vi "气密封测试.vi"() -> ()   [LabVIEW 2014]
uses:
  <vilib>/Instr/_visa.llb/VISA Flush IO Buffer Mask.ctl
  <vilib>/Utility/config.llb/NI_LVConfig.lvlib
  <vilib>/Utility/config.llb/Write Key (String).vi
  <vilib>/Utility/miscctls.llb/LVRowAndColumnTypeDef.ctl
  <vilib>/Utility/config.llb/Read Key (String).vi
  <vilib>/Instr/_visa.llb/VISA Configure Serial Port (Instr).vi
panel:
  in  "右扫码启动":bool
  in  "左扫码启动":bool
  in  "错误输入（无错误） 2":errorcluster caption="错误输入（无错误）"
  out "错误输出 4":errorcluster caption="错误输出"
  out "错误输出 3":errorcluster caption="错误输出"
  in  "错误输入（无错误）":errorcluster
  out "合格 2":bool
  out "StepCode 2":u16
  out "Ready 2":bool
  out "右合格":bool
  out "替换数量 2":i32
  out "结果 2":string
  in  "合格次数 2":u16
  out "泄漏单位 2":string
  out "压力单位 2":string
  in  "检测次数 2":u16
  in  "合格状态右":dbl=2.0
  out "StatusResults 2":u16 format="%b"
  out "LeakUnit 2":u16(ring) items=["ml/min"=51000, "cm3/s"=0, "cm3/min"=1000, "cm3/h"=2000, "mm3/h"=3000, "CalibartedPascal"=4000, "Pa"=6000, "Bar"=11000, "Kpa"=12000, "PSI"=13000, "Mbar"=14000, "Mpa"=15000, "Inch3/s"=46000, "Inch3/min"=47000, "Inch3/hour"=48000]
  out "PressureUnit 2":u16(ring) items=["cm3/s"=0, "cm3/min"=1000, "cm3/h"=2000, "mm3/h"=3000, "CalibartedPascal"=4000, "Pa"=6000, "Bar"=11000, "Kpa"=12000, "PSI"=13000, "Mbar"=14000, "Mpa"=15000, "Inch3/s"=46000, "Inch3/min"=47000, "Inch3/hour"=48000]
  out "ProgramNumber 2":u16
  out "结果压力 2":dbl
  out "结果漏率 2":dbl
  out "扫码信息 B":string
  out "开始启动仪器 2":bool
  out "开始启动仪器":bool
  in  "扫码选程序":bool=TRUE
  out "错误输出":errorcluster
  out "写入的字节":i32
  out "数值 2":i32
  in  "扫码流程":dbl
  out "左合格":bool
  out "合格":bool
  in  "合格次数":u16
  in  "检测次数":u16
  out "扫码信息A":string
  out "结果漏率":dbl
  out "结果压力":dbl
  out "替换数量":i32
  out "ATEQ程序号-1":i32
  in  "扫码关键词":u16(ring)
  in  "启动仪器":dbl
  out "ProgramNumber":u16
  in  "选项卡控件":enum32{"主页面", "设置"}(tab)
  in  "扫码开/关B":bool
  in  "扫码开/关A":bool
  in  "选择检验员B":u16(ring) items=["李红", "", "", "", "", "", "", "", "", "", "", "", "", "", "", "", "", "", "", "", "", "", "", "", "", "", "", "", "", "", "", "", "", "", ""]
  in  "选择产品型号B":u16(ring) items=["EV80", "E109", "", "", "", "", "", "", "", "", "", "", "", "", "", "", "", "", "", "", "", "", "", "", "", "", "", "", "", "", "", "", "", "", ""]
  in  "单腔/双腔A":bool
  out "最终结果A":bool
  in  "选择检验员A":u16(ring) items=["李红", "", "", "", "", "", "", "", "", "", "", "", "", "", "", "", "", "", "", "", "", "", "", "", "", "", "", "", "", "", "", "", "", "", ""]
  out "实时压力A":dbl
  out "实时漏率A":dbl
  in  "确定修改A":bool
  out "当前序号A":string
  in  "序号清零A":bool
  in  "修改当前序号A":string
  out "显示表格":string[][](table)
  in  "选择产品型号A":u16(ring) items=["EV80", "E109", "", "", "", "", "", "", "", "", "", "", "", "", "", "", "", "", "", "", "", "", "", "", "", "", "", "", "", "", "", "", "", "", ""]
  out "程序号":i32
  out "二维码A":string
  out "二维码B":string
  out "实时压力B":dbl
  out "实时漏率B":dbl
  out "最终结果B":bool
  in  "单腔/双腔B":bool
  in  "修改当前序号B":string
  in  "确定修改B":bool
  in  "序号清零B":bool
  out "当前序号B":string
  in  "表格控件":string[][](table)
  in  "确定按钮":bool
  in  "活动单元格:活动单元格":T1
  out "泄漏单位":string
  out "压力单位":string
  out "PressureUnit":u16(ring) items=["cm3/s"=0, "cm3/min"=1000, "cm3/h"=2000, "mm3/h"=3000, "CalibartedPascal"=4000, "Pa"=6000, "Bar"=11000, "Kpa"=12000, "PSI"=13000, "Mbar"=14000, "Mpa"=15000, "Inch3/s"=46000, "Inch3/min"=47000, "Inch3/hour"=48000]
  out "StatusResults":u16 format="%b"
  out "LeakUnit":u16(ring) items=["ml/min"=51000, "cm3/s"=0, "cm3/min"=1000, "cm3/h"=2000, "mm3/h"=3000, "CalibartedPascal"=4000, "Pa"=6000, "Bar"=11000, "Kpa"=12000, "PSI"=13000, "Mbar"=14000, "Mpa"=15000, "Inch3/s"=46000, "Inch3/min"=47000, "Inch3/hour"=48000]
  in  "合格状态左":dbl
  out "Ready":bool
  out "StepCode":u16
  out "结果":string
  # "气密性检测设备"
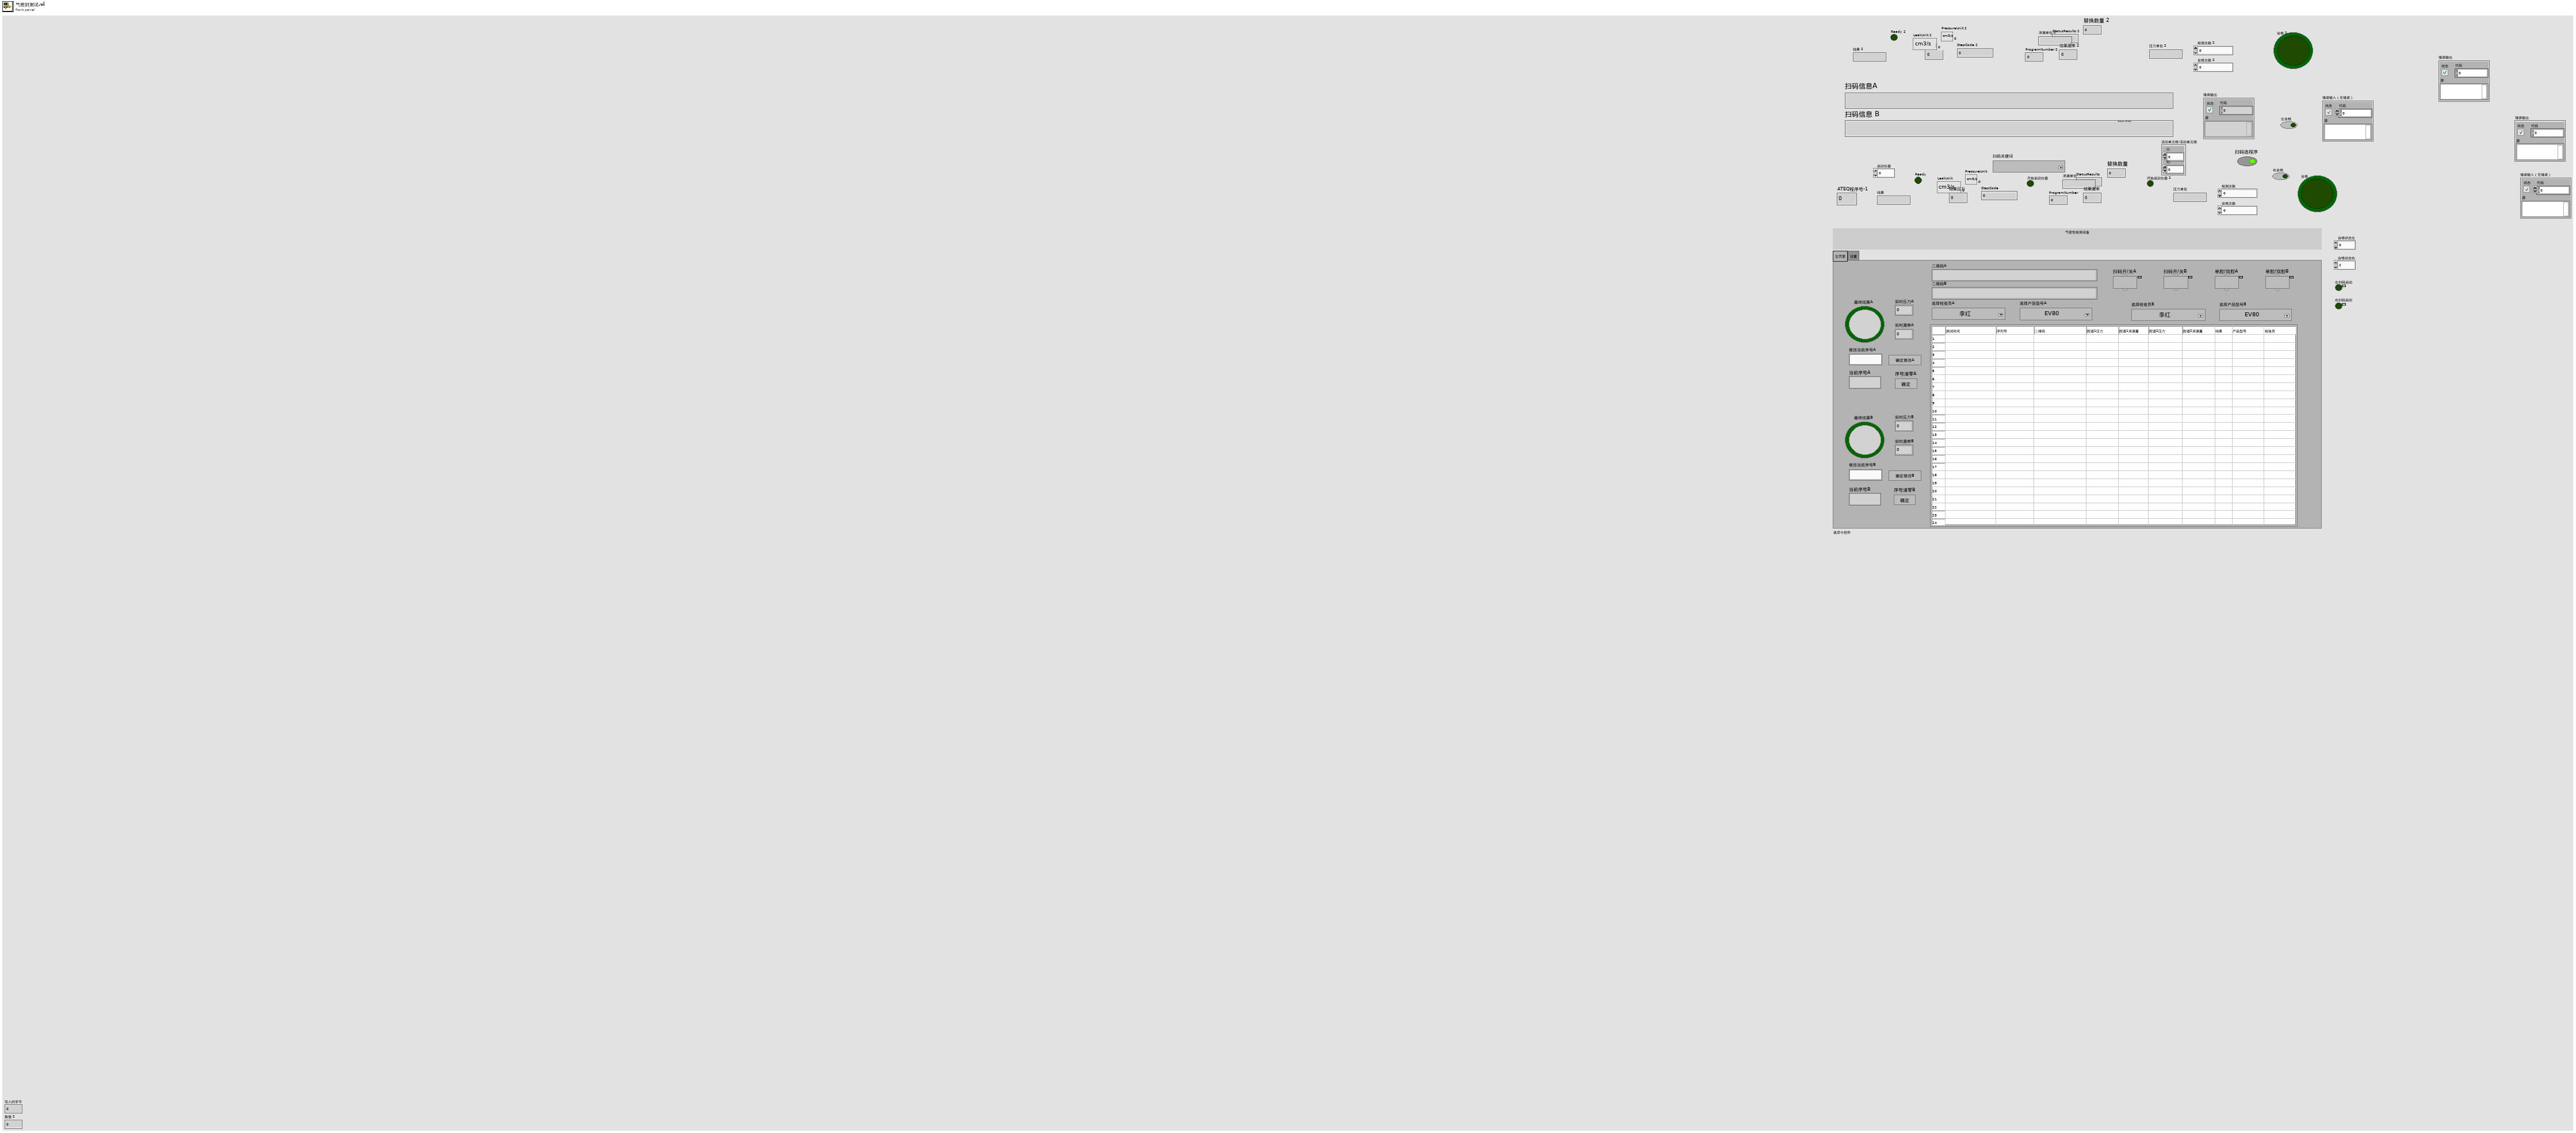
[diagram p1: front panel]
types:
  T1 = typedef "LVRowAndColumnTypeDef.ctl" = cluster{"Row":i32, "Column":i32}
  T2 = enum16{"Init", "Loop", "Write LOFF", "Write LON", "Read", "Exit", "Open", "Close"}
  T3 = typedef "NI_LVConfig.lvlib/Config Data RefNum.ctl" = refnum<k1>
  T4 = enum8{"Enabled", "Disabled", "Disabled and Grayed Out"}
  T5 = typedef "VISA Flush IO Buffer Mask.ctl" = u16
  T6 = enum16{"Standard", "Buffered", "CRLF", "Immediate"}
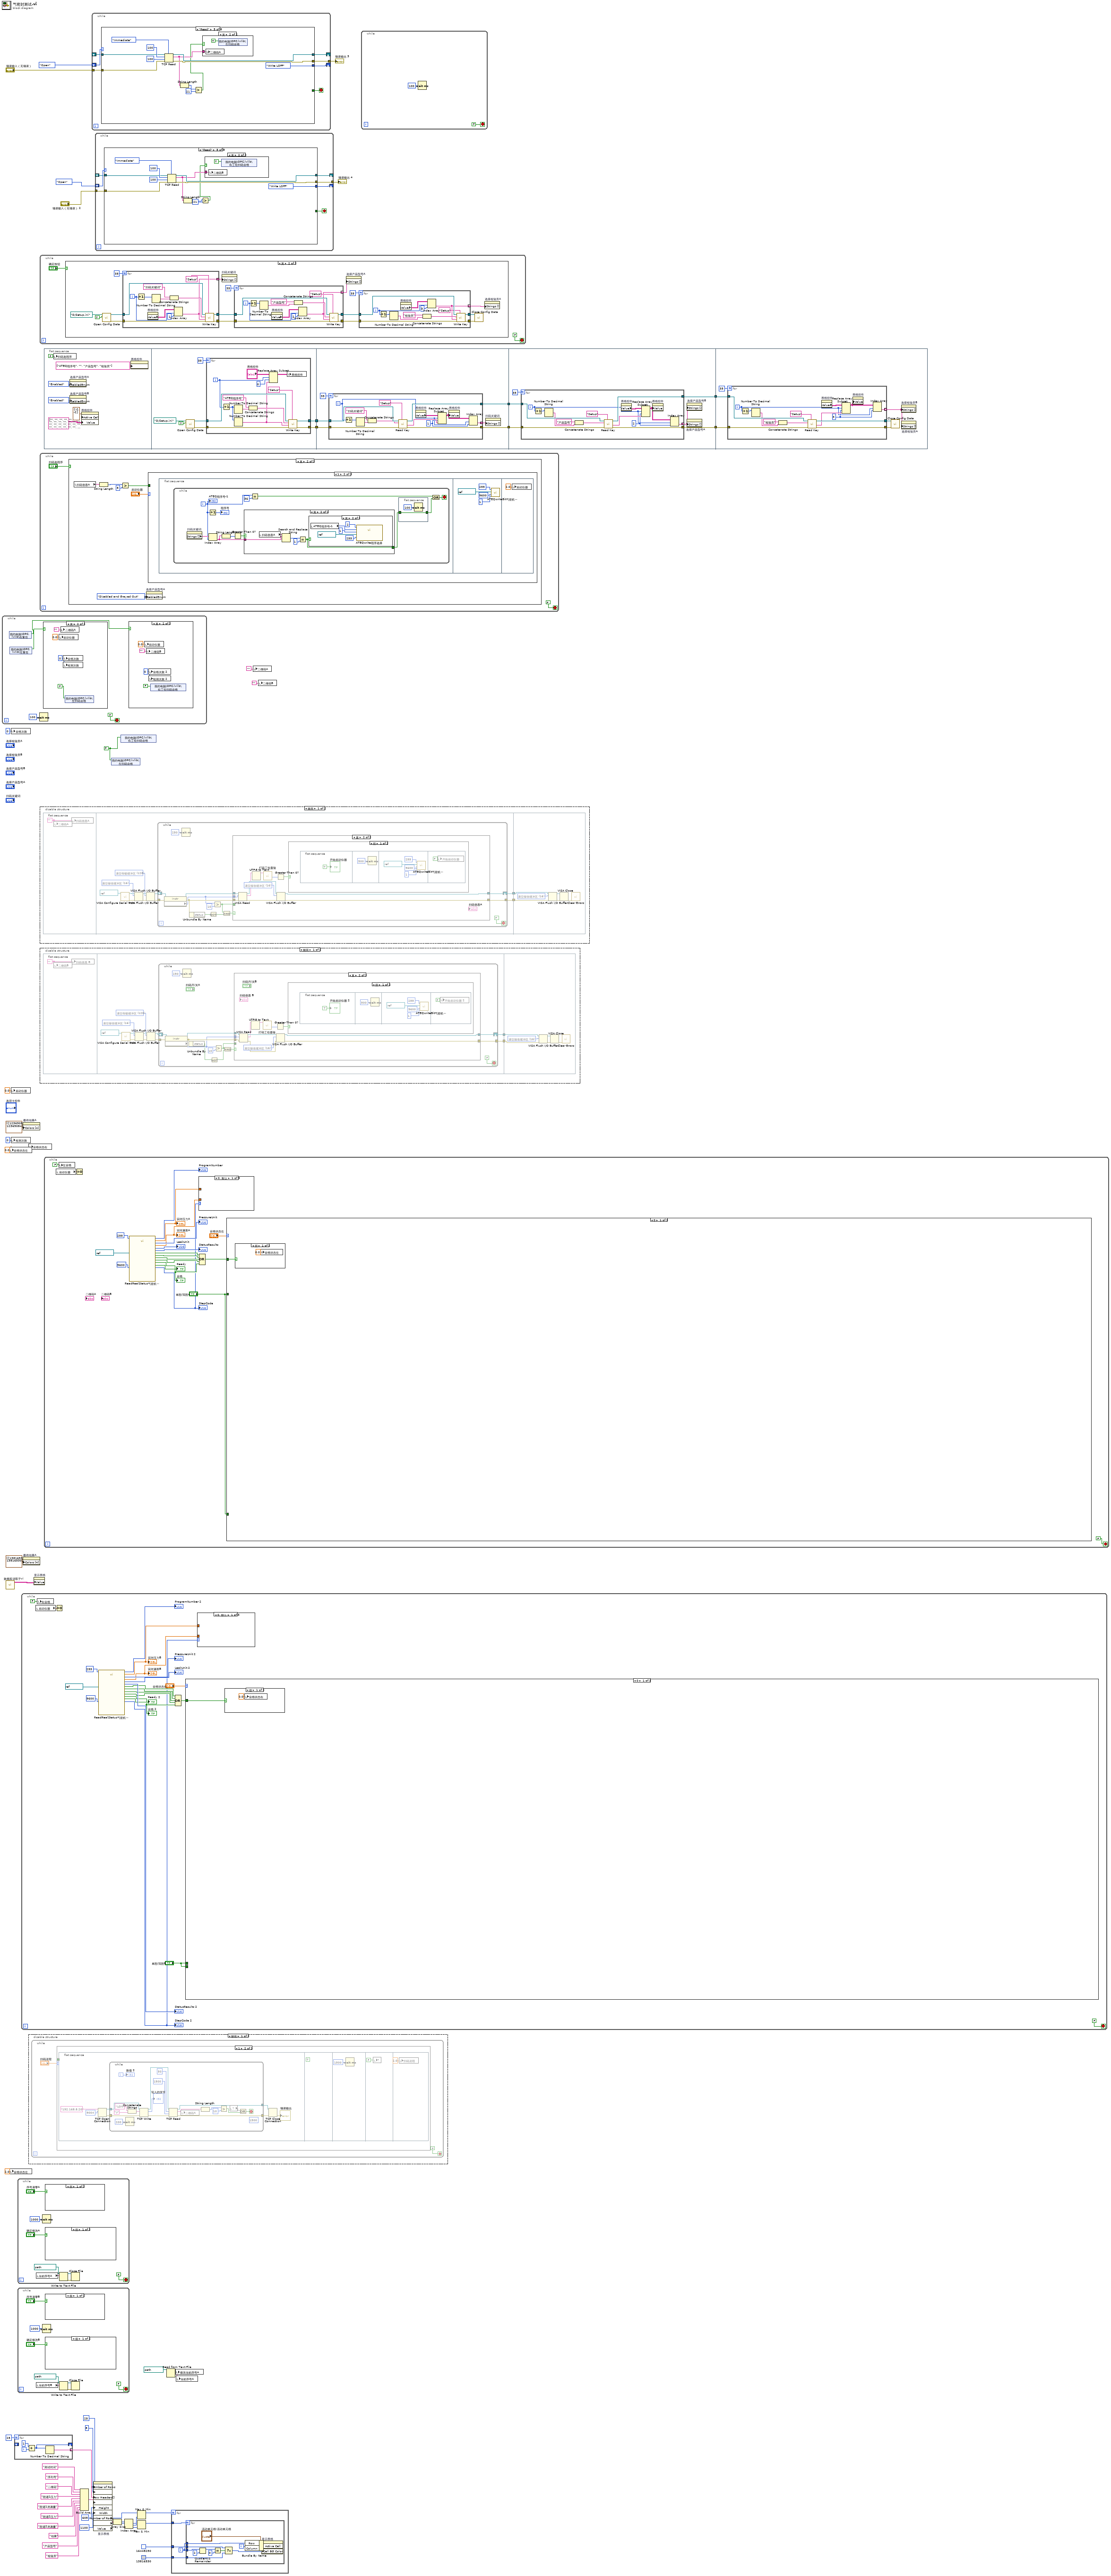
[diagram p0: block diagram]
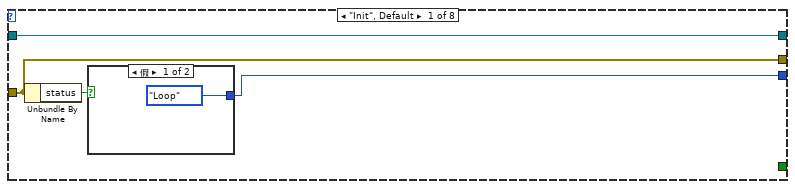
[diagram p2: hidden frame]
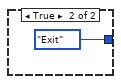
[diagram p3: hidden frame]
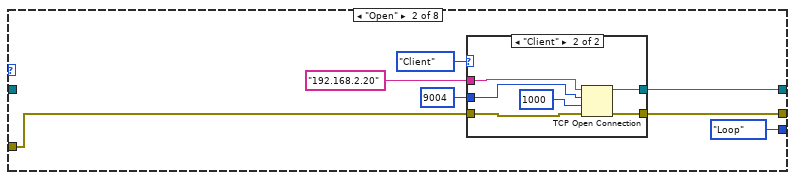
[diagram p4: hidden frame]
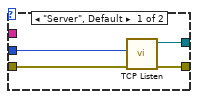
[diagram p5: hidden frame]
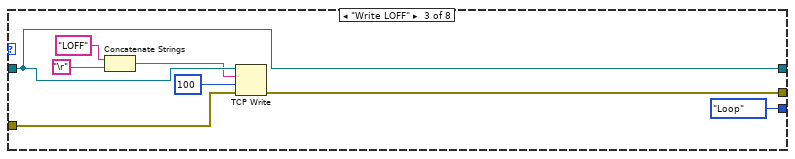
[diagram p6: hidden frame]
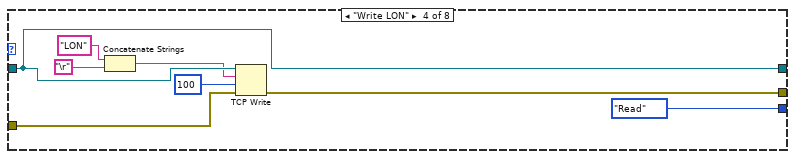
[diagram p7: hidden frame]
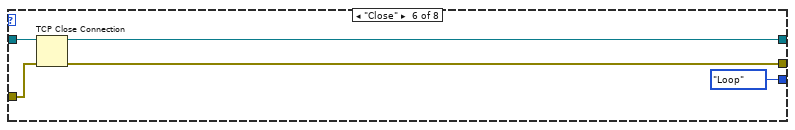
[diagram p9: hidden frame]
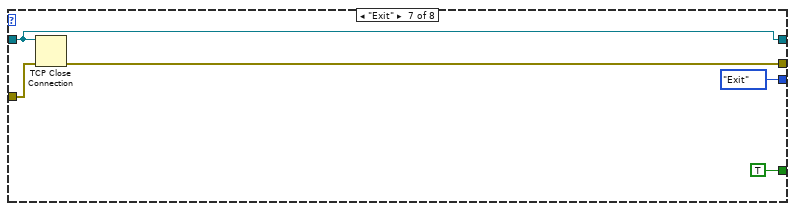
[diagram p10: hidden frame]
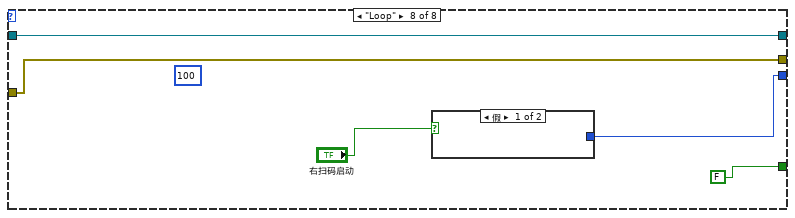
[diagram p11: hidden frame]
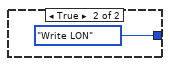
[diagram p12: hidden frame]
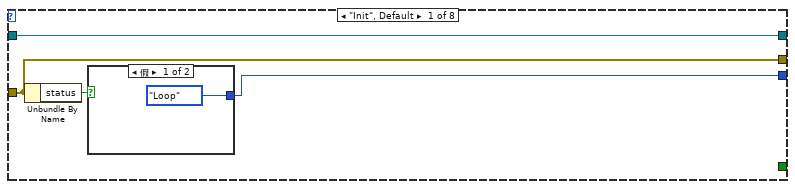
[diagram p13: hidden frame]
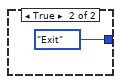
[diagram p14: hidden frame]
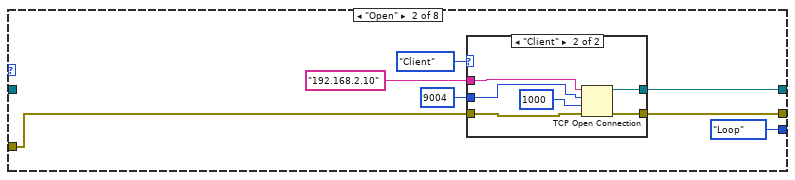
[diagram p15: hidden frame]
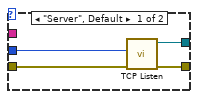
[diagram p16: hidden frame]
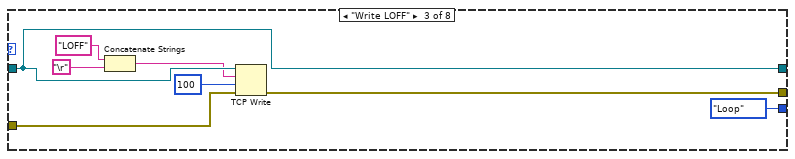
[diagram p17: hidden frame]
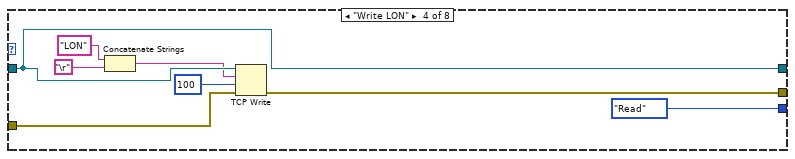
[diagram p18: hidden frame]
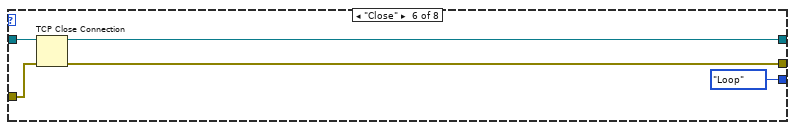
[diagram p20: hidden frame]
diagram:
  w3 = FALSE ("左扫码合格")
  w4 = 0.0 ("合格状态")
  n1 = while {
    stop <- FALSE stop-if-true
    n2 = shared-variable "我的电脑\\OPC.lvlib\\右复位"() -> (w53:bool)  [unwired: 1 in, 1 out]
    n3 = shared-variable "我的电脑\\OPC.lvlib\\左复位"() -> (w54:bool)  [unwired: 1 in, 1 out]
    n4 = Wait (ms)(milliseconds to wait=u32 100 ("等待时间（毫秒）")) -> ()  [unwired: 1 out]
    n5 = case shown="真" w54 {
      frame False {
      }
      frame True {
        w62 = u16 0 ("合格次数")
        n6 = local write "启动仪器"(0.0 ("启动仪器")) -> ()
        n7 = local write "二维码A"("") -> ()
        n8 = local write "合格次数"(w62) -> ()
        n9 = local write "检测次数"(w62) -> ()
        n10 = shared-variable "我的电脑\\OPC.lvlib\\左扫码合格"(FALSE ("左扫码合格")) -> ()  [unwired: 1 in, 1 out]
      }
    }
    n11 = case shown="真" w53 {
      frame False {
      }
      frame True {
        w60 = u16 0 ("合格次数")
        n12 = local write "启动仪器"(0.0 ("启动仪器")) -> ()
        n13 = local write "二维码B"("") -> ()
        n14 = local write "合格次数 2"(w60) -> ()
        n15 = local write "检测次数 2"(w60) -> ()
        n16 = shared-variable "我的电脑\\OPC.lvlib\\右工位扫码合格"(FALSE ("左扫码合格")) -> ()  [unwired: 1 in, 1 out]
      }
    }
  }
  n17 = call "数据库读取子vi.vi"() -> ("Data"=w16:string[][])  [unwired: 11 in]
  n18 = local write "合格状态左"(w4) -> ()
  n19 = local write "合格状态左"(2.0 ("合格状态")) -> ()
  n20 = local write "合格次数"(u16 0 ("合格次数")) -> ()
  n21 = local write "启动仪器"(0.0 ("启动仪器")) -> ()
  n22 = local write "检测次数"(u16 0 ("检测次数")) -> ()
  n23 = for {
    N: 25 -> [_]
    shift-right: [w66] -> _
    shift-left: _ -> [_]
    tunnel: [w65] -> w43 mode=indexing
    i -> [w67]
    n24 = Add(x=1, y=w67) -> (x+y=w66:i32)
    n25 = Number To Decimal String(number=w66) -> (decimal integer string=w65:string)  [unwired: 1 in]
  }
  n26 = while {
    stop <- FALSE stop-if-true
    n27 = local read "当前序号A"() -> (w71:string)
    n28 = Wait (ms)(milliseconds to wait=u32 1000 ("等待时间（毫秒）")) -> ()  [unwired: 1 out]
    n29 = case shown="假" "序号清零A" {
      frame False {
      }
      frame True {
        n30 = call "序号清零子vi.vi"() -> ("当日序号"=→"当前序号A":string)  [unwired: 11 in]
      }
    }
    n31 = case shown="假" "确定修改A" {
      frame False {
      }
      frame True {
        n32 = local write "当前序号A"("修改当前序号A") -> ()
        n33 = Write to Text File(file (use dialog)=path "D:/序号.txt" ("文件（使用对话框）"), text="修改当前序号A") -> (refnum out=w79:refnum<file>, error out=w80:errorcluster)  [unwired: 2 in, 1 out]
        n34 = Close File(refnum=w79, error in=w80) -> ()  [unwired: 2 out]
      }
    }
    n35 = Write to Text File(file (use dialog)=path "D:/序号A.txt" ("文件（使用对话框）"), text=w71) -> (refnum out=w72:refnum<file>, error out=w73:errorcluster)  [unwired: 2 in, 1 out]
    n36 = Close File(refnum=w72, error in=w73) -> ()  [unwired: 2 out]
  }
  n37 = while {
    stop <- FALSE stop-if-true
    n38 = local read "当前序号B"() -> (w84:string)
    n39 = Wait (ms)(milliseconds to wait=u32 1000 ("等待时间（毫秒）")) -> ()  [unwired: 1 out]
    n40 = case shown="假" "序号清零B" {
      frame False {
      }
      frame True {
        n41 = call "序号清零子vi.vi"() -> ("当日序号"=→"当前序号B":string)  [unwired: 11 in]
      }
    }
    n42 = case shown="假" "确定修改B" {
      frame False {
      }
      frame True {
        n43 = local write "当前序号B"("修改当前序号B") -> ()
        n44 = Write to Text File(file (use dialog)=path "D:/序号B.txt" ("文件（使用对话框）"), text="修改当前序号B") -> (refnum out=w92:refnum<file>, error out=w93:errorcluster)  [unwired: 2 in, 1 out]
        n45 = Close File(refnum=w92, error in=w93) -> ()  [unwired: 2 out]
      }
    }
    n46 = Write to Text File(file (use dialog)=path "D:/序号B.txt" ("文件（使用对话框）"), text=w84) -> (refnum out=w85:refnum<file>, error out=w86:errorcluster)  [unwired: 2 in, 1 out]
    n47 = Close File(refnum=w85, error in=w86) -> ()  [unwired: 2 out]
  }
  n48 = while {
    stop <- FALSE stop-if-true
    n49 = local read "启动仪器"() -> (w98:dbl)
    n50 = local write "右合格"(FALSE) -> ()
    n51 = Equal To 0?(x=w98) -> ()  [unwired: 1 out]
    n52 = call "ReadRealStatus气密机一.vi"("从站地址"=u8 255, "VISA"=refnum<visa-resource-name> "COM7", "baud rate"=u32 9600) -> ("Ready"=→"Ready 2":bool, "Pass"=w106:bool, "StepCode"=w103:u16, "ProgramNumber"=→"ProgramNumber 2":u16, "Pressure"=w101:dbl, "PressureUnit"=→"PressureUnit 2":u16, "AL"=w107:bool, "Leak"=w102:dbl, "PressureAL"=w108:bool, "RD"=w109:bool, "TD"=w105:bool, "StatusResults"=→"StatusResults 2":u16, "LeakUnit"=→"LeakUnit 2":u16)
    "合格 2" <- w106
    "StepCode 2" <- w103
    "实时漏率B" <- w102
    "实时压力B" <- w101
    n53 = Compound Arithmetic op=OR ("复合运算")(w105, w109, w108, w107, w106) -> (w110:bool)
    n54 = case shown="0" "合格状态右" {
      tunnel: w110 -> [w120 _ w323]
      tunnel: "单腔/双腔B" -> [_ w124 _]
      tunnel: "单腔/双腔B" -> [_ w123 _]
      frame 0 {
        n55 = case shown="假" w120 {
          frame False {
            n56 = local write "合格状态右"(0.0 ("合格状态")) -> ()
          }
          frame True {
            n57 = local write "合格状态右"(1.0 ("合格状态")) -> ()
          }
        }
      }
      frame 1 {
        n58 = flat-sequence {
          tunnel: [w130] -> w127
          tunnel: [w131] -> w125
          tunnel: w124 -> [w131]
          tunnel: w123 -> [w130]
          tunnel: [w138] -> w129
          tunnel: [w137] -> w128
          tunnel: w127 -> [w137]
          tunnel: [w136] -> w126
          tunnel: w125 -> [w136]
          tunnel: w129 -> [w161]
          tunnel: w128 -> [w159]
          tunnel: w126 -> [w158]
          frame #0 {
            n59 = local write "最终结果B"(FALSE ("最终结果")) -> ()
            n60 = property on="最终结果B" class="Bool (严格)"("Colors [4]"=cluster{u32, u32}[] [{13816530, 13816530}] ("颜色[4]")) -> ()  [unwired: 2 in, 2 out]
            n61 = Increment(x="检测次数 2") -> (x+1=w134:u16)
            n62 = local write "检测次数 2"(w134) -> ()
          }
          frame #1 {
            n63 = local read "合格 2"() -> (w138:bool)
            n64 = property on="PressureUnit 2" class="Ring (严格)"() -> ("Value"=w140:u16)  [unwired: 2 in, 2 out]
            n65 = property on="LeakUnit 2" class="Ring (严格)"() -> ("Value"=w139:u16)  [unwired: 2 in, 2 out]
            n66 = Wait (ms)(milliseconds to wait=u32 200 ("等待时间（毫秒）")) -> ()  [unwired: 1 out]
            n67 = case shown="真" w138 {
              frame False {
                n68 = local write "结果 2"("NG" ("结果")) -> ()
              }
              frame True {
                n69 = Increment(x="合格次数 2") -> (x+1=w155:u16)
                n70 = local write "合格次数 2"(w155) -> ()
                "结果 2" <- "OK" ("结果")
              }
            }
            n71 = case shown="8000" w139 {
              frame 0, Default {
              }
              frame 1000 {
                n72 = local write "泄漏单位 2"("cm3/min" ("压力单位")) -> ()
              }
              frame 2000 {
                n73 = local write "泄漏单位 2"("ml/h" ("压力单位")) -> ()
              }
              frame 6000 {
                "泄漏单位 2" <- "pa"
              }
              frame 7000 {
                n74 = local write "泄漏单位 2"("pa") -> ()
              }
              frame 8000 {
                n75 = local write "泄漏单位 2"("pa/s" ("泄漏单位")) -> ()
              }
              frame 9000 {
                n76 = local write "泄漏单位 2"("pa/s" ("泄漏单位")) -> ()
              }
              frame 51000 {
                n77 = local write "泄漏单位 2"("ml/min" ("压力单位")) -> ()
              }
            }
            n78 = case shown="15000" w140 {
              frame 0, Default {
              }
              frame 11000 {
                n79 = local write "压力单位 2"("Bar" ("压力单位")) -> ()
              }
              frame 12000 {
                n80 = local write "压力单位 2"("Kpa" ("压力单位")) -> ()
              }
              frame 13000 {
                n81 = local write "压力单位 2"("Psi" ("压力单位")) -> ()
              }
              frame 14000 {
                n82 = local write "压力单位 2"("mbar" ("压力单位")) -> ()
              }
              frame 15000 {
                "压力单位 2" <- "Mpa"
              }
            }
          }
          frame #2 {
            n83 = local read "检测次数 2"() -> (w160:u16)
            n84 = local read "当前序号B"() -> (w162:string)
            n85 = local write "修改当前序号B"(w162) -> ()
            n86 = case shown="2" w160 {
              tunnel: w161 -> [_ w166 w244]
              tunnel: w159 -> [_ w164 _]
              tunnel: w158 -> [_ w163 _]
              frame 0, Default {
              }
              frame 1 {
                n87 = flat-sequence {
                  tunnel: [w168] -> w167
                  tunnel: w166 -> [w168]
                  tunnel: w167 -> [w173]
                  tunnel: [w171] -> w165
                  tunnel: w164 -> [w172]
                  tunnel: w163 -> [w171]
                  tunnel: w165 -> [w233]
                  frame #0 {
                    n88 = call "序号加一子vi.vi"() -> ("当日序号"=w169:string)  [unwired: 11 in]
                    n89 = local write "当前序号B"(w169) -> ()
                  }
                  frame #1 {
                    n90 = property on="选择检验员B" class="Ring (严格)"() -> ("Strings []"=w201:string[], "Value"=w202:u16)  [unwired: 2 in, 2 out]
                    n91 = case shown="假" w173 {
                      tunnel: [w222 w225] -> w204
                      tunnel: [w221 w226] -> w205
                      frame False {
                        n92 = local read "实时漏率B"() -> (w220:dbl)
                        n93 = Equal To 0?(x=w220) -> (x = 0?=w219:bool)
                        n94 = case shown="真" w219 {
                          tunnel: [w223 99999.0] -> w222
                          frame False {
                            n95 = local read "实时漏率B"() -> (w223:dbl)
                          }
                          frame True {
                          }
                        }
                        n96 = local read "实时压力B"() -> (w221:dbl)
                      }
                      frame True {
                        n97 = local read "结果漏率 2"() -> (w225:dbl)
                        n98 = local read "结果压力 2"() -> (w226:dbl)
                      }
                    }
                    n99 = case shown="真" w173 {
                      tunnel: [w210 w214] -> w174
                      tunnel: w172 -> [w209 w213]
                      frame False {
                        n100 = case shown="假" w209 {
                          tunnel: ["NG" ("结果") _] -> w210
                          frame False {
                            n101 = property on="最终结果B" class="Bool (严格)"("Colors [4]"=cluster{u32, u32}[] [{16711680, 16711680}] ("颜色[4]")) -> ()  [unwired: 2 in, 2 out]
                          }
                          frame True {
                          }
                        }
                      }
                      frame True {
                        n102 = case shown="真" w213 {
                          tunnel: ["OK" ("结果") _] -> w214
                          frame False {
                            n103 = local write "最终结果B"(TRUE ("最终结果")) -> ()
                            n104 = property on="最终结果B" class="Bool (严格)"("Colors [4]"=cluster{u32, u32}[] [{6618880, 6618880}] ("颜色[4]")) -> ()  [unwired: 2 in, 2 out]
                          }
                          frame True {
                            n105 = property on="最终结果B" class="Bool (严格)"("Colors [4]"=cluster{u32, u32}[] [{13816530, 13816530}] ("颜色[4]")) -> ()  [unwired: 2 in, 2 out]
                          }
                        }
                      }
                    }
                    n106 = local read "ProgramNumber 2"() -> (w197:u16)
                    n107 = Index Array(array=w201, index=w202) -> ()  [unwired: 1 out]
                    n108 = Number To Decimal String(number=w197, width (-)=i16 3 ("宽度(-)")) -> (decimal integer string=w198:string)
                    n109 = call <vilib>:"Space Constant.vi"() -> ("String"=w199:string)
                    n110 = Search and Replace String(replace all?=TRUE ("替换全部？(F)"), input string=w198, search string=w199, replace string="0" ("替换字符串(\"\")")) -> (number of replacements=→"替换数量 2":i32)  [unwired: 4 in, 3 out]
                    n111 = local read "扫码选程序"() -> (w203:bool)
                    n112 = case shown="假" w203 {
                      tunnel: [w227 w231] -> w208
                      frame False {
                        n113 = property on="选择产品型号B" class="Ring (严格)"() -> ("Strings []"=w228:string[], "Value"=w229:u16)  [unwired: 2 in, 2 out]
                        n114 = Index Array(array=w228, index=w229) -> (element=w227:string)
                      }
                      frame True {
                        n115 = local read "ATEQ程序号-1"() -> (w230:i32)
                        n116 = property on="选择产品型号A" class="Ring (严格)"() -> ("Strings []"=w232:string[])  [unwired: 2 in, 2 out]
                        n117 = Index Array(array=w232, index=w230) -> (element=w231:string)
                      }
                    }
                    n118 = local read "当前序号B"() -> (w196:string)
                    n119 = Format Date/Time String(time format string (%c)="%Y%m%d" ("时间格式字符串(%c)")) -> (date/time string=w190:string)  [unwired: 2 in]
                    n120 = local read "泄漏单位 2"() -> (w194:string)
                    n121 = local read "压力单位 2"() -> (w193:string)
                    n122 = Write to Text File(file (use dialog)=path "d:/序号B.txt" ("文件（使用对话框）"), text=w196) -> ()  [unwired: 2 in, 3 out]
                    n123 = Number To Fractional String(number=w204, width (-)=i16 5 ("宽度(-)"), precision (6)=i16 2 ("精度(6)")) -> (F-format string=w192:string)  [unwired: 1 in]
                    n124 = Number To Fractional String(number=w205, width (-)=i16 6 ("宽度(-)"), precision (6)=i16 2 ("精度(6)")) -> (F-format string=w191:string)  [unwired: 1 in]
                    n125 = Concatenate Strings(w190, w196, "B" ("时间格式字符串(%c)")) -> (w206:string)
                    n126 = Concatenate Strings(w192, w194) -> (w207:string)
                    n127 = Concatenate Strings(w191, w193) -> (w176:string)
                    n128 = Format Date/Time String(time format string (%c)="%Y/%m/%d %H:%M:%S" ("时间格式字符串(%c)")) -> (date/time string=w195:string)  [unwired: 2 in]
                    n129 = local read "二维码B"() -> (w175:string)
                    n130 = Write to Text File(file (use dialog)=path "d:/检测时间B.txt" ("文件（使用对话框）"), text=w195) -> ()  [unwired: 2 in, 3 out]
                    n131 = Write to Text File(file (use dialog)=path "d:/腔道1泄漏量B.txt" ("文件（使用对话框）"), text=w207) -> ()  [unwired: 2 in, 3 out]
                    n132 = Write to Text File(file (use dialog)=path "d:/腔道1压力B.txt" ("文件（使用对话框）"), text=w176) -> ()  [unwired: 2 in, 3 out]
                    n133 = call "数据库保存子vi.vi"("#1 Pressure"=w176, "Part No."=w208, "Result"=w174, "2D Code"=w175, "#1 Leakage"=w207, "Serial No."=w206, "Time"=w195) -> ()  [unwired: 5 in]
                  }
                  frame #2 {
                    n134 = case shown="假" w233 {
                      frame False {
                        w234 = u16 0 ("合格次数")
                        n135 = local write "检测次数 2"(w234) -> ()
                        n136 = local write "合格次数 2"(w234) -> ()
                      }
                      frame True {
                      }
                    }
                  }
                }
              }
              frame 2 {
                n137 = flat-sequence {
                  tunnel: w244 -> [w273]
                  tunnel: [w257] -> w243
                  tunnel: [w256] -> w242
                  tunnel: [w246] -> w241
                  tunnel: [w255] -> w240
                  tunnel: [w254] -> w239
                  tunnel: [w253] -> w238
                  tunnel: [w252] -> w237
                  tunnel: [w251] -> w236
                  tunnel: [w250] -> w235
                  tunnel: w243 -> [w310]
                  tunnel: w242 -> [w311]
                  tunnel: w241 -> [w308]
                  tunnel: w240 -> [w306]
                  tunnel: w239 -> [w304]
                  tunnel: w238 -> [w302]
                  tunnel: w237 -> [w300]
                  tunnel: w236 -> [w298]
                  tunnel: w235 -> [w296]
                  frame #0 {
                    n138 = case shown="假" w273 {
                      tunnel: [w291 w294] -> w280
                      tunnel: [w290 w295] -> w281
                      frame False {
                        n139 = local read "实时漏率B"() -> (w289:dbl)
                        n140 = Equal To 0?(x=w289) -> (x = 0?=w288:bool)
                        n141 = case shown="假" w288 {
                          tunnel: [w292 99999.0] -> w291
                          frame False {
                            n142 = local read "实时漏率B"() -> (w292:dbl)
                          }
                          frame True {
                          }
                        }
                        n143 = local read "实时压力B"() -> (w290:dbl)
                      }
                      frame True {
                        n144 = local read "结果漏率 2"() -> (w294:dbl)
                        n145 = local read "结果压力 2"() -> (w295:dbl)
                      }
                    }
                    n146 = local read "合格次数 2"() -> (w249:u16)
                    n147 = Equal?(x=w249, y=u16 2) -> (x = y?=w247:bool)
                    n148 = case shown="真" w247 {
                      tunnel: ["NG" "OK"] -> w246
                      frame False {
                        n149 = property on="最终结果B" class="Bool (严格)"("Colors [4]"=cluster{u32, u32}[] [{16711680, 16711680}] ("颜色[4]")) -> ()  [unwired: 2 in, 2 out]
                        "最终结果B" <- FALSE ("最终结果")
                      }
                      frame True {
                        w286 = TRUE ("最终结果")
                        n150 = property on="最终结果B" class="Bool (严格)"("Colors [4]"=cluster{u32, u32}[] [{6618880, 6618880}] ("颜色[4]")) -> ()  [unwired: 2 in, 2 out]
                        n151 = local write "最终结果B"(w286) -> ()
                        "右合格" <- w286
                      }
                    }
                    n152 = local read "泄漏单位 2"() -> (w278:string)
                    n153 = local read "压力单位 2"() -> (w277:string)
                    n154 = local read "当前序号B"() -> (w279:string)
                    n155 = Format Date/Time String(time format string (%c)="%Y%m%d" ("时间格式字符串(%c)")) -> (date/time string=w274:string)  [unwired: 2 in]
                    n156 = Number To Fractional String(number=w280, width (-)=i16 5 ("宽度(-)"), precision (6)=i16 2 ("精度(6)")) -> (F-format string=w276:string)  [unwired: 1 in]
                    n157 = Number To Fractional String(number=w281, width (-)=i16 6 ("宽度(-)"), precision (6)=i16 2 ("精度(6)")) -> (F-format string=w275:string)  [unwired: 1 in]
                    n158 = Write to Text File(file (use dialog)=path "d:/序号B.txt" ("文件（使用对话框）"), text=w279) -> ()  [unwired: 2 in, 3 out]
                    n159 = Concatenate Strings(w274, w279, "B" ("字符串")) -> (w251:string)
                    n160 = Concatenate Strings(w276, w278) -> (w252:string)
                    n161 = Concatenate Strings(w275, w277) -> (w253:string)
                    n162 = call "数据库插入子vi.vi"("result"=w246, "2_Leakage"=w252, "2_Pressure"=w253, "Serial_No"=w251) -> ()  [unwired: 8 in]
                    n163 = Write to Text File(file (use dialog)=path "d:/腔道2泄漏量B.txt" ("文件（使用对话框）"), text=w252) -> ()  [unwired: 2 in, 3 out]
                    n164 = Write to Text File(file (use dialog)=path "d:/腔道2压力B.txt" ("文件（使用对话框）"), text=w253) -> ()  [unwired: 2 in, 3 out]
                    n165 = property on="选择产品型号B" class="Ring (严格)"() -> ("Strings []"=w260:string[], "Value"=w261:u16)  [unwired: 2 in, 2 out]
                    n166 = property on="选择检验员B" class="Ring (严格)"() -> ("Strings []"=w258:string[], "Value"=w259:u16)  [unwired: 2 in, 2 out]
                    n167 = Index Array(array=w260, index=w261) -> (element=w256:string)
                    n168 = Index Array(array=w258, index=w259) -> (element=w250:string)
                    n169 = Read from Text File(file (use dialog)=path "d:/检测时间B.txt" ("文件（使用对话框）")) -> (text=w257:string)  [unwired: 3 in, 3 out]
                    n170 = Read from Text File(file (use dialog)=path "d:/腔道2压力B.txt" ("文件（使用对话框）")) -> (text=w255:string)  [unwired: 3 in, 3 out]
                    n171 = Read from Text File(file (use dialog)=path "d:/腔道1泄漏量B.txt" ("文件（使用对话框）")) -> (text=w254:string)  [unwired: 3 in, 3 out]
                  }
                  frame #1 {
                    n172 = call <vilib>:"Space Constant.vi"() -> ("String"=w312:string)
                    n173 = call <vilib>:"Space Constant.vi"() -> ("String"=w309:string)
                    n174 = call <vilib>:"Space Constant.vi"() -> ("String"=w305:string)
                    n175 = call <vilib>:"Space Constant.vi"() -> ("String"=w301:string)
                    n176 = call <vilib>:"Space Constant.vi"() -> ("String"=w297:string)
                    n177 = Wait (ms)(milliseconds to wait=u32 1000 ("等待时间（毫秒）")) -> ()  [unwired: 1 out]
                    n178 = Concatenate Strings(w311, w312, w310, w309, w308, "\n", w306, w305, w304, "\n", w302, w301, w300, "\n", w298, w297, w296) -> (w314:string)
                    n179 = Write to Text File(file (use dialog)=path "d:/激光打码B.txt" ("文件（使用对话框）"), text=w314) -> ()  [unwired: 2 in, 3 out]
                  }
                  frame #2 {
                    w316 = u16 0 ("合格次数")
                    n180 = local write "检测次数 2"(w316) -> ()
                    n181 = local write "合格次数 2"(w316) -> ()
                  }
                }
              }
            }
          }
          frame #3 {
            n182 = call <vilib>:"Space Constant.vi"() -> ("String"=w319:string)
            n183 = local write "二维码B"(w319) -> ()
            n184 = Write to Text File(file (use dialog)=path "d:/扫码结果B.txt" ("文件（使用对话框）"), text=w319) -> ()  [unwired: 2 in, 3 out]
            n185 = call "数据库读取子vi.vi"() -> ("Data"=w317:string[][])  [unwired: 11 in]
            n186 = local write "显示表格"(w317) -> ()
          }
          frame #4 {
            n187 = Wait (ms)(milliseconds to wait=u32 2000 ("等待时间（毫秒）")) -> ()  [unwired: 1 out]
          }
          frame #5 {
            n188 = local write "右合格"(FALSE) -> ()
          }
          frame #6 {
            n189 = local write "合格状态右"(2.0) -> ()
          }
        }
      }
      frame 2, Default {
        n190 = case shown="真" w323 {
          frame False {
            n191 = local write "合格状态右"(0.0 ("合格状态")) -> ()
          }
          frame True {
          }
        }
      }
    }
    n192 = case shown="0, 默认" w103 {
      tunnel: w102 -> [_ _ w119]
      tunnel: w101 -> [_ _ w118]
      frame 0, Default {
      }
      frame 1 {
        n193 = property on="最终结果B" class="Bool (严格)"("Colors [4]"=cluster{u32, u32}[] [{12369084, 12369084}] ("颜色[4]")) -> ()  [unwired: 2 in, 2 out]
      }
      frame 6 {
        "结果压力 2" <- w118
        "结果漏率 2" <- w119
      }
    }
  }
  n194 = property on="最终结果A" class="Bool (严格)"("Colors [4]"=cluster{u32, u32}[] [{12369084, 12369084}] ("颜色[4]")) -> ()  [unwired: 2 in, 2 out]
  n195 = property on="最终结果A" class="Bool (严格)"("Colors [4]"=cluster{u32, u32}[] [{13816530, 13816530}] ("颜色[4]")) -> ()  [unwired: 2 in, 2 out]
  n196 = disable-structure shown="禁用" {
    frame Disabled {
      n197 = while {
        stop <- FALSE stop-if-true
        n198 = case shown="1" "扫码流程" {
          tunnel: [w328 _ w361] -> w326
          frame 0, Default {
            n199 = case shown="真" w328 {
              frame False {
              }
              frame True {
                n200 = local write "扫码流程"(1.0 ("扫码流程")) -> ()
              }
            }
          }
          frame 1 {
            n201 = flat-sequence {
              frame #0 {
                n202 = TCP Open Connection(address="192.168.8.20" ("地址"), remote port or service name=u16 9004 ("远程端口或服务名称")) -> (connection ID=w333:refnum<k5>, error out=w334:errorcluster)  [unwired: 3 in]
                n203 = while {
                  tunnel: w333 -> [w355]
                  tunnel: [w348] -> w332
                  tunnel: w334 -> [w356]
                  tunnel: [w347] -> w331
                  i -> [w343]
                  stop <- w338 stop-if-true
                  (unwired) 1500 ("超时毫秒(25000)")
                  n204 = Wait (ms)(milliseconds to wait=u32 200 ("等待时间（毫秒）")) -> ()  [unwired: 1 out]
                  n205 = Concatenate Strings("LON", "\r") -> (w352:string)
                  n206 = TCP Write(connection ID=w355, data in=w352, error in (no error)=w356) -> (connection ID out=w351:refnum<k5>, bytes written=→"写入的字节":i32, error out=w350:errorcluster)  [unwired: 1 in]
                  n207 = TCP Read(connection ID=w351, bytes to read=50 ("读取的字节"), error in (no error)=w350, 9:1500 ("超时毫秒(25000)")) -> (connection ID out=w348:refnum<k5>, data out=w337:string, error out=w347:errorcluster)  [unwired: 1 in]
                  n208 = local write "二维码A"(w337) -> ()
                  n209 = String Length(string=w337) -> (length=w342:i32)
                  n210 = Greater?(x=w342, y=10) -> (0:w340:bool)
                  n211 = local read item#-1() -> (w339)
                  n212 = Or(x=w339, y=w340) -> (x .or. y?=w338:bool)
                  "数值 2" <- w343
                }
                n213 = TCP Close Connection(connection ID=w332, error in (no error)=w331) -> (error out=→"错误输出":errorcluster)  [unwired: 1 in, 1 out]
              }
              frame #1 {
                w357 = TRUE ("扫码完成")
              }
              frame #2 {
                n214 = Wait (ms)(milliseconds to wait=u32 1500 ("等待时间（毫秒）")) -> ()  [unwired: 1 out]
              }
              frame #3 {
                n215 = local write item#-1(FALSE ("扫码完成")) -> ()
              }
              frame #4 {
                n216 = local write "扫码流程"(2.0 ("扫码流程")) -> ()
              }
            }
          }
          frame 2 {
            n217 = case shown="假" w361 {
              frame False {
                n218 = local write "扫码流程"(0.0 ("扫码流程")) -> ()
              }
              frame True {
              }
            }
          }
        }
      }
    }
    frame Enabled {
    }
  }
  n219 = local write "合格状态右"(w4) -> ()
  n220 = property on="显示表格" class="Tbl (严格)"("Value"=w16) -> ()  [unwired: 2 in, 2 out]
  n221 = while {
    stop <- FALSE stop-if-true
    n222 = case shown="真" "确定按钮" {
      frame False {
      }
      frame True {
        n223 = call <vilib>:"Open Config Data.vi"("create file if necessary (T)"=TRUE, "configuration file path"=path "D:/Setup.ini") -> ("error out"=w376:errorcluster, "refnum"=w379:T3)  [unwired: 7 in, 1 out]
        n224 = for {
          N: 35 -> [_]
          tunnel: w379 -> [w419]
          tunnel: [w415] -> w373
          tunnel: w376 -> [w414]
          tunnel: [w413] -> w372
          tunnel: [w407] -> w365 mode=indexing
          i -> [w412]
          n225 = Increment(x=w412) -> (x+1=w410:i32)
          n226 = property on="表格控件" class="Tbl (严格)"() -> ("Value"=w417:string[][])  [unwired: 2 in, 2 out]
          n227 = Number To Decimal String(number=w410) -> (decimal integer string=w409:string)  [unwired: 1 in]
          n228 = Concatenate Strings("扫码关键词" ("字符串"), w409) -> (w408:string)
          n229 = Index Array(array=w417, index (row)=w412, index (col)=1 ("Column")) -> (element=w407:string)
          n230 = call-poly <vilib>:"Write Key.vi"("section"="Setup", "error in (no error)"=w414, "value"=w407, "key"=w408, "refnum"=w419) -> ("error out"=w413:errorcluster, "refnum out"=w415:T3)  [unwired: 4 in, 1 out]
        }
        n231 = property on="扫码关键词" class="Ring (严格)"("Strings []"=w365) -> ()  [unwired: 2 in, 2 out]
        n232 = for {
          N: 35 -> [_]
          tunnel: w373 -> [w406]
          tunnel: [w402] -> w371
          tunnel: w372 -> [w401]
          tunnel: [w400] -> w370
          tunnel: [w394] -> w367 mode=indexing
          i -> [w399]
          n233 = Increment(x=w399) -> (x+1=w397:i32)
          n234 = Number To Decimal String(number=w397) -> (decimal integer string=w396:string)  [unwired: 1 in]
          n235 = property on="表格控件" class="Tbl (严格)"() -> ("Value"=w404:string[][])  [unwired: 2 in, 2 out]
          n236 = Concatenate Strings("产品型号" ("字符串"), w396) -> (w395:string)
          n237 = Index Array(array=w404, index (row)=w399, index (col)=2 ("Column")) -> (element=w394:string)
          n238 = call-poly <vilib>:"Write Key.vi"("section"="Setup", "error in (no error)"=w401, "value"=w394, "key"=w395, "refnum"=w406) -> ("error out"=w400:errorcluster, "refnum out"=w402:T3)  [unwired: 4 in, 1 out]
        }
        n239 = property on="选择产品型号A" class="Ring (严格)"("Strings []"=w367) -> ()  [unwired: 2 in, 2 out]
        n240 = for {
          N: 35 -> [_]
          tunnel: w371 -> [w393]
          tunnel: [w389] -> w369
          tunnel: w370 -> [w388]
          tunnel: [w387] -> w368
          tunnel: [w381] -> w366 mode=indexing
          i -> [w386]
          n241 = Increment(x=w386) -> (x+1=w384:i32)
          n242 = Number To Decimal String(number=w384) -> (decimal integer string=w383:string)  [unwired: 1 in]
          n243 = property on="表格控件" class="Tbl (严格)"() -> ("Value"=w391:string[][])  [unwired: 2 in, 2 out]
          n244 = Concatenate Strings("检验员" ("字符串"), w383) -> (w382:string)
          n245 = Index Array(array=w391, index (row)=w386, index (col)=3 ("Column")) -> (element=w381:string)
          n246 = call-poly <vilib>:"Write Key.vi"("section"="Setup", "error in (no error)"=w388, "value"=w381, "key"=w382, "refnum"=w393) -> ("error out"=w387:errorcluster, "refnum out"=w389:T3)  [unwired: 4 in, 1 out]
        }
        n247 = call <vilib>:"Close Config Data.vi"("error in (no error)"=w368, "refnum"=w369) -> ()  [unwired: 8 in, 2 out]
        n248 = property on="选择检验员A" class="Ring (严格)"("Strings []"=w366) -> ()  [unwired: 2 in, 2 out]
      }
    }
  }
  n249 = while {
    stop <- FALSE stop-if-true
    n250 = case shown="真" "扫码选程序" {
      frame False {
        n251 = disable-structure shown="启用" {
          frame Disabled {
            n252 = event shown="[1] \"选择产品型号A\": 值改变" {
              selector: _ -> [_ _]
              dyn-events: _ -> [_ _]
              timeout: 100 -> [_ _]
              event Timeout {
                n253 = event-data() -> ()  [unwired: 1 in, 3 out]
              }
              event "选择产品型号A": Value Change {
                n254 = event-data() -> ("NewVal"=w425:u16)  [unwired: 1 in, 5 out]
                n255 = Increment(x=w425) -> (x+1=w424:u16)
                n256 = local write "程序号"(w424) -> ()
                n257 = call "ATEQwrite程序选择.vi"("VISA resource name"=refnum<visa-resource-name> "COM4", "从站地址"=u8 255, "The number of write"=u16 1, "实际程序号-1"=w425, "Write Address"=u16 2) -> ()  [unwired: 6 in, 1 out]
              }
            }
          }
          frame Enabled {
          }
        }
        n258 = property on="选择产品型号A" class="Ring (严格)"("DisabledEnum"=T4."Enabled" ("禁用")) -> ()  [unwired: 2 in, 2 out]
      }
      frame True {
        n259 = local read "扫码信息A"() -> (w435:string)
        n260 = String Length(string=w435) -> (length=w434:i32)
        n261 = Greater?(x=w434, y=8) -> (0:w431:bool)
        n262 = property on="选择产品型号A" class="Ring (严格)"("DisabledEnum"=T4."Disabled and Grayed Out" ("禁用")) -> ()  [unwired: 2 in, 2 out]
        n263 = case shown="1" "启动仪器" {
          tunnel: w431 -> [w436 _ w466]
          frame 0, Default {
            n264 = case shown="真" w436 {
              frame False {
              }
              frame True {
                n265 = local write "启动仪器"(1.0 ("启动仪器")) -> ()
              }
            }
          }
          frame 1 {
            n266 = flat-sequence {
              frame #0 {
                n267 = while {
                  i -> [w442]
                  stop <- w438 stop-if-true
                  n268 = property on="扫码关键词" class="Ring (严格)"() -> ("Strings []"=w448:string[])  [unwired: 2 in, 2 out]
                  n269 = Increment(x=w442) -> (x+1=→"程序号":i32)
                  n270 = Index Array(array=w448, index=w442) -> (element=w443:string)
                  n271 = String Length(string=w443) -> (length=w447:i32)
                  n272 = Greater Than 0?(x=w447) -> (x > 0?=w446:bool)
                  n273 = case shown="真" w446 {
                    tunnel: [_ w452] -> w445
                    tunnel: w443 -> [_ w451]
                    frame False {
                    }
                    frame True {
                      n274 = local read "扫码信息A"() -> (w454:string)
                      n275 = Search and Replace String(input string=w454, search string=w451) -> (number of replacements=w455:i32)  [unwired: 6 in, 3 out]
                      n276 = Equal?(x=w455, y=1) -> (x = y?=w452:bool)
                      n277 = case shown="真" w452 {
                        frame False {
                        }
                        frame True {
                          n278 = local read "ATEQ程序号-1"() -> (w457:i32)
                          n279 = call "ATEQwrite程序选择.vi"("VISA resource name"=refnum<visa-resource-name> "COM4", "从站地址"=u8 255, "The number of write"=u16 1, "实际程序号-1"=w457, "Write Address"=u16 2) -> ()  [unwired: 6 in, 1 out]
                        }
                      }
                    }
                  }
                  n280 = Equal?(x=w442, y=36) -> (x = y?=w440:bool)
                  n281 = flat-sequence {
                    tunnel: [w449] -> w439
                    tunnel: w445 -> [w449]
                    frame #0 {
                      n282 = Wait (ms)(milliseconds to wait=u32 100 ("等待时间（毫秒）")) -> ()  [unwired: 1 out]
                    }
                  }
                  n283 = Compound Arithmetic op=OR ("复合运算")(w440, w439) -> (w438:bool)
                  "ATEQ程序号-1" <- w442
                }
              }
              frame #1 {
                n284 = call "ATEQwriteBit气密机一.vi"("Write Address"=u16 1, "baud rate"=u32 9600, "VISA resource name"=refnum<visa-resource-name> "COM4", "从站地址"=u8 255) -> ()  [unwired: 7 in, 1 out]
              }
              frame #2 {
                n285 = local write "启动仪器"(2.0 ("启动仪器")) -> ()
              }
            }
          }
          frame 2 {
            n286 = case shown="假" w466 {
              frame False {
                n287 = local write "启动仪器"(0.0 ("启动仪器")) -> ()
              }
              frame True {
              }
            }
          }
        }
      }
    }
  }
  n288 = disable-structure shown="禁用" {
    frame Disabled {
      n289 = flat-sequence {
        tunnel: [w481] -> w469
        tunnel: [w480] -> w468
        tunnel: w469 -> [w531]
        tunnel: w468 -> [w532]
        frame #0 {
          w470 = ""
          n290 = local write "二维码A"(w470) -> ()
          n291 = local write "扫码信息A"(w470) -> ()
        }
        frame #1 {
          w472 = T5 128 items=["清空接收缓冲区"=16, "向设备写入传输缓冲区"=32, "清空接收缓冲区（无I/O）"=64, "清空传输缓冲区"=128] ("Mask")
          w475 = T5 16 items=["清空接收缓冲区"=16, "向设备写入传输缓冲区"=32, "清空接收缓冲区（无I/O）"=64, "清空传输缓冲区"=128] ("Mask")
          n292 = call-poly "VISA Configure Serial Port"("VISA resource name"=refnum<visa-resource-name> "COM6") -> ("VISA resource name out"=w476:refnum<visa-resource-name>, "error out"=w477:errorcluster)  [unwired: 6 in, 7 out]
          n293 = VISA Flush I/O Buffer(VISA resource name=w476, mask (16)=w475, error in (no error)=w477) -> (VISA resource name out=w474:refnum<visa-resource-name>, error out=w473:errorcluster)
          n294 = VISA Flush I/O Buffer(VISA resource name=w474, mask (16)=w472, error in (no error)=w473) -> (VISA resource name out=w479:refnum<visa-resource-name>, error out=w478:errorcluster)
          n295 = while {
            tunnel: w478 -> [w494]
            tunnel: [w493] -> w481
            shift-right: [w492] -> w480
            shift-left: w479 -> [w495]
            stop <- FALSE ("关闭") stop-if-true
            n296 = property class="Instr"(reference=w495, error in=w494) -> (reference out=w491:refnum<visa-resource-name>, error out=w490:errorcluster, "Serial Settings:Number of Bytes at Serial Port"=w488:u32)
            n297 = Wait (ms)(milliseconds to wait=u32 250 ("等待时间（毫秒）")) -> ()  [unwired: 1 out]
            n298 = Unbundle By Name(w490) -> ("status"=w482:bool)
            n299 = Not(x=w482) -> (.not. x?=w487:bool)
            n300 = Greater?(x=w488, y=u32 10) -> (0:w486:bool)
            n301 = And(x=w486, y=w487) -> (x .and. y?=w485:bool)
            n302 = case shown="真" w485 {
              tunnel: [w499 w513] -> w493
              tunnel: [w500 w515] -> w492
              tunnel: w491 -> [w498 w519]
              tunnel: w490 -> [w497 w518]
              tunnel: w488 -> [_ w517]
              tunnel: w486 -> [w496 _]
              frame False {
                n303 = case shown="真" w496 {
                  tunnel: [w502 w507] -> w500
                  tunnel: [w501 w506] -> w499
                  tunnel: w498 -> [w502 w505]
                  tunnel: w497 -> [w501 w504]
                  frame False {
                  }
                  frame True {
                    w503 = T5 16 items=["清空接收缓冲区"=16, "向设备写入传输缓冲区"=32, "清空接收缓冲区（无I/O）"=64, "清空传输缓冲区"=128] ("Mask")
                    n304 = VISA Flush I/O Buffer(VISA resource name=w505, mask (16)=w503, error in (no error)=w504) -> (VISA resource name out=w507:refnum<visa-resource-name>, error out=w506:errorcluster)
                  }
                }
              }
              frame True {
                w512 = T5 16 items=["清空接收缓冲区"=16, "向设备写入传输缓冲区"=32, "清空接收缓冲区（无I/O）"=64, "清空传输缓冲区"=128] ("Mask")
                n305 = VISA Read(VISA resource name=w519, byte count=w517, error in (no error)=w518) -> (VISA resource name out=w516:refnum<visa-resource-name>, read buffer=w509:string, error out=w514:errorcluster)  [unwired: 1 out]
                n306 = UTF-8 to Text(11:w509) -> (3:w508:string)  [unwired: 2 in, 1 out]
                n307 = call "打码工位查验.vi"("二维码"=w508) -> ("Rows Fetched"=w511:i32)  [unwired: 9 in, 1 out]
                n308 = Greater Than 0?(x=w511) -> (x > 0?=w510:bool)
                n309 = VISA Flush I/O Buffer(VISA resource name=w516, mask (16)=w512, error in (no error)=w514) -> (VISA resource name out=w515:refnum<visa-resource-name>, error out=w513:errorcluster)
                n310 = case shown="假" w510 {
                  frame False {
                    n311 = flat-sequence {
                      frame #0 {
                        "开始启动仪器" <- TRUE ("开始启动仪器")
                      }
                      frame #1 {
                        n312 = Wait (ms)(milliseconds to wait=u32 500 ("等待时间（毫秒）")) -> ()  [unwired: 1 out]
                      }
                      frame #2 {
                        n313 = call "ATEQwriteBit气密机一.vi"("Write Address"=u16 1, "baud rate"=u32 9600, "VISA resource name"=refnum<visa-resource-name> "COM3", "从站地址"=u8 255) -> ()  [unwired: 7 in, 1 out]
                      }
                      frame #3 {
                        n314 = local write "开始启动仪器"(FALSE ("开始启动仪器")) -> ()
                      }
                    }
                  }
                  frame True {
                    n315 = One Button Dialog(message="重复扫码" ("消息")) -> ()  [unwired: 1 in, 1 out]
                  }
                }
              }
            }
          }
        }
        frame #2 {
          w529 = T5 16 items=["清空接收缓冲区"=16, "向设备写入传输缓冲区"=32, "清空接收缓冲区（无I/O）"=64, "清空传输缓冲区"=128] ("Mask")
          n316 = VISA Flush I/O Buffer(VISA resource name=w532, mask (16)=w529, error in (no error)=w531) -> (VISA resource name out=w530:refnum<visa-resource-name>, error out=w528:errorcluster)
          n317 = VISA Close(VISA resource name=w530, error in (no error)=w528) -> (error out=w533:errorcluster)
          n318 = call <vilib>:"Clear Errors.vi"("error in (no error)"=w533) -> ()  [unwired: 5 in, 2 out]
        }
      }
    }
    frame Enabled {
    }
  }
  n319 = disable-structure shown="禁用" {
    frame Disabled {
      n320 = flat-sequence {
        tunnel: [w547] -> w535
        tunnel: [w546] -> w534
        tunnel: w535 -> [w597]
        tunnel: w534 -> [w598]
        frame #0 {
          w536 = ""
          n321 = local write "二维码B"(w536) -> ()
          n322 = local write "扫码信息 B"(w536) -> ()
        }
        frame #1 {
          w538 = T5 128 items=["清空接收缓冲区"=16, "向设备写入传输缓冲区"=32, "清空接收缓冲区（无I/O）"=64, "清空传输缓冲区"=128] ("Mask")
          w541 = T5 16 items=["清空接收缓冲区"=16, "向设备写入传输缓冲区"=32, "清空接收缓冲区（无I/O）"=64, "清空传输缓冲区"=128] ("Mask")
          n323 = call-poly "VISA Configure Serial Port"("VISA resource name"=refnum<visa-resource-name> "COM8") -> ("VISA resource name out"=w542:refnum<visa-resource-name>, "error out"=w543:errorcluster)  [unwired: 6 in, 7 out]
          n324 = VISA Flush I/O Buffer(VISA resource name=w542, mask (16)=w541, error in (no error)=w543) -> (VISA resource name out=w540:refnum<visa-resource-name>, error out=w539:errorcluster)
          n325 = VISA Flush I/O Buffer(VISA resource name=w540, mask (16)=w538, error in (no error)=w539) -> (VISA resource name out=w545:refnum<visa-resource-name>, error out=w544:errorcluster)
          n326 = while {
            tunnel: w544 -> [w560]
            tunnel: [w559] -> w547
            shift-right: [w558] -> w546
            shift-left: w545 -> [w561]
            stop <- FALSE ("关闭") stop-if-true
            n327 = property class="Instr"(reference=w561, error in=w560) -> (reference out=w557:refnum<visa-resource-name>, error out=w556:errorcluster, "Serial Settings:Number of Bytes at Serial Port"=w554:u32)
            n328 = Wait (ms)(milliseconds to wait=u32 250 ("等待时间（毫秒）")) -> ()  [unwired: 1 out]
            n329 = Unbundle By Name(w556) -> ("status"=w548:bool)
            n330 = Not(x=w548) -> (.not. x?=w553:bool)
            n331 = Greater?(x=w554, y=u32 10) -> (0:w552:bool)
            n332 = And(x=w552, y=w553) -> (x .and. y?=w551:bool)
            n333 = case shown="真" w551 {
              tunnel: [w565 w579] -> w559
              tunnel: [w566 w581] -> w558
              tunnel: w557 -> [w564 w585]
              tunnel: w556 -> [w563 w584]
              tunnel: w554 -> [_ w583]
              tunnel: w552 -> [w562 _]
              frame False {
                n334 = case shown="真" w562 {
                  tunnel: [w568 w573] -> w566
                  tunnel: [w567 w572] -> w565
                  tunnel: w564 -> [w568 w571]
                  tunnel: w563 -> [w567 w570]
                  frame False {
                  }
                  frame True {
                    w569 = T5 16 items=["清空接收缓冲区"=16, "向设备写入传输缓冲区"=32, "清空接收缓冲区（无I/O）"=64, "清空传输缓冲区"=128] ("Mask")
                    n335 = VISA Flush I/O Buffer(VISA resource name=w571, mask (16)=w569, error in (no error)=w570) -> (VISA resource name out=w573:refnum<visa-resource-name>, error out=w572:errorcluster)
                  }
                }
              }
              frame True {
                w578 = T5 16 items=["清空接收缓冲区"=16, "向设备写入传输缓冲区"=32, "清空接收缓冲区（无I/O）"=64, "清空传输缓冲区"=128] ("Mask")
                n336 = VISA Read(VISA resource name=w585, byte count=w583, error in (no error)=w584) -> (VISA resource name out=w582:refnum<visa-resource-name>, read buffer=w575:string, error out=w580:errorcluster)  [unwired: 1 out]
                n337 = UTF-8 to Text(11:w575) -> (3:w574:string)  [unwired: 2 in, 1 out]
                n338 = call "打码工位查验.vi"("二维码"=w574) -> ("Rows Fetched"=w577:i32)  [unwired: 9 in, 1 out]
                n339 = Greater Than 0?(x=w577) -> (x > 0?=w576:bool)
                n340 = VISA Flush I/O Buffer(VISA resource name=w582, mask (16)=w578, error in (no error)=w580) -> (VISA resource name out=w581:refnum<visa-resource-name>, error out=w579:errorcluster)
                n341 = case shown="假" w576 {
                  frame False {
                    n342 = flat-sequence {
                      frame #0 {
                        "开始启动仪器 2" <- TRUE ("开始启动仪器")
                      }
                      frame #1 {
                        n343 = Wait (ms)(milliseconds to wait=u32 500 ("等待时间（毫秒）")) -> ()  [unwired: 1 out]
                      }
                      frame #2 {
                        n344 = call "ATEQwriteBit气密机一.vi"("Write Address"=u16 1, "baud rate"=u32 9600, "VISA resource name"=refnum<visa-resource-name> "COM7", "从站地址"=u8 255) -> ()  [unwired: 7 in, 1 out]
                      }
                      frame #3 {
                        n345 = local write "开始启动仪器 2"(FALSE ("开始启动仪器")) -> ()
                      }
                    }
                  }
                  frame True {
                    n346 = One Button Dialog(message="重复扫码" ("消息")) -> ()  [unwired: 1 in, 1 out]
                  }
                }
              }
            }
          }
        }
        frame #2 {
          w595 = T5 16 items=["清空接收缓冲区"=16, "向设备写入传输缓冲区"=32, "清空接收缓冲区（无I/O）"=64, "清空传输缓冲区"=128] ("Mask")
          n347 = VISA Flush I/O Buffer(VISA resource name=w598, mask (16)=w595, error in (no error)=w597) -> (VISA resource name out=w596:refnum<visa-resource-name>, error out=w594:errorcluster)
          n348 = VISA Close(VISA resource name=w596, error in (no error)=w594) -> (error out=w599:errorcluster)
          n349 = call <vilib>:"Clear Errors.vi"("error in (no error)"=w599) -> ()  [unwired: 5 in, 2 out]
        }
      }
    }
    frame Enabled {
    }
  }
  n350 = flat-sequence {
    tunnel: [w607] -> w25
    tunnel: [w606] -> w24
    tunnel: w25 -> [w631]
    tunnel: w24 -> [w630]
    tunnel: [w629] -> w23
    tunnel: [w628] -> w22
    tunnel: w23 -> [w652]
    tunnel: w22 -> [w651]
    tunnel: [w650] -> w21
    tunnel: [w649] -> w20
    tunnel: w21 -> [w673]
    tunnel: w20 -> [w672]
    frame #0 {
      n351 = local write "扫码选程序"(FALSE ("扫码选程序")) -> ()
      n352 = property on="选择产品型号A" class="Ring (严格)"("DisabledEnum"=T4."Enabled" ("禁用")) -> ()  [unwired: 2 in, 2 out]
      n353 = property on="选择产品型号B" class="Ring (严格)"("DisabledEnum"=T4."Enabled" ("禁用")) -> ()  [unwired: 2 in, 2 out]
      n354 = property on="表格控件" class="Tbl (严格)"("Active Cell"=T1 {"Row"=-2, "Column"=-2} ("活动单元格:活动单元格"), "Value"=string[][] [["", "", "", ""], ["", "", "", ""], ["", "", "", ""], ["", "", "", ""], ["", "", "", ""], ["", "", "", ""], ["", "", "", ""], ["", "", "", ""], ["", "", "", ""], ["", "", "", ""], ["", "", "", ""], ["", "", "", ""], ["", "", "", ""], ["", "", "", ""], ["", "", "", ""], ["", "", "", ""], ["", "", "", ""], ["", "", "", ""], ["", "", "", ""], ["", "", "", ""], ["", "", "", ""], ["", "", "", ""], ["", "", "", ""], ["", "", "", ""], ["", "", "", ""], ["", "", "", ""], ["", "", "", ""], ["", "", "", ""], ["", "", "", ""], ["", "", "", ""], ["", "", "", ""], ["", "", "", ""], ["", "", "", ""], ["", "", "", ""], ["", "", "", ""], ["", "", "", ""], ["", "", "", ""], ["", "", "", ""], ["", "", "", ""], ["", "", "", ""], ["", "", "", ""], ["", "", "", ""], ["", "", "", ""], ["", "", "", ""], ["", "", "", ""], ["", "", "", ""], ["", "", "", ""], ["", "", "", ""], ["", "", "", ""], ["", "", "", ""], ["", "", "", ""], ["", "", "", ""], ["", "", "", ""], ["", "", "", ""], ["", "", "", ""], ["", "", "", ""], ["", "", "", ""], ["", "", "", ""], ["", "", "", ""], ["", "", "", ""], ["", "", "", ""], ["", "", "", ""], ["", "", "", ""], ["", "", "", ""], ["", "", "", ""], ["", "", "", ""], ["", "", "", ""], ["", "", "", ""], ["", "", "", ""], ["", "", "", ""], ["", "", "", ""], ["", "", "", ""], ["", "", "", ""], ["", "", "", "0"]] ("表格控件")) -> ()  [unwired: 2 in, 2 out]
      n355 = property on="表格控件" class="Tbl (严格)"("Column Headers[]"=string[] ["ATEQ程序号", "", "产品型号", "检验员"] ("列首字符串[]")) -> ()  [unwired: 2 in, 2 out]
    }
    frame #1 {
      n356 = call <vilib>:"Open Config Data.vi"("create file if necessary (T)"=TRUE, "configuration file path"=path "D:/Setup.ini") -> ("error out"=w612:errorcluster, "refnum"=w609:T3)  [unwired: 7 in, 1 out]
      n357 = for {
        N: 35 -> [_]
        tunnel: w609 -> [w626]
        tunnel: [w624] -> w607
        tunnel: w612 -> [w623]
        tunnel: [w622] -> w606
        i -> [w616]
        n358 = Increment(x=w616) -> (x+1=w618:i32)
        n359 = Number To Decimal String(number=w618) -> (decimal integer string=w620:string)  [unwired: 1 in]
        n360 = Number To Decimal String(number=w618) -> (decimal integer string=w615:string)  [unwired: 1 in]
        n361 = Concatenate Strings("ATEQ程序号" ("字符串"), w620) -> (w619:string)
        n362 = Replace Array Subset(array="表格控件", new element=w615, index (row)=w616, index (col)=0 ("索引 (列)")) -> (w614:string[][])
        n363 = local write "表格控件"(w614) -> ()
        n364 = call-poly <vilib>:"Write Key.vi"("section"="Setup", "error in (no error)"=w623, "value"=w615, "key"=w619, "refnum"=w626) -> ("error out"=w622:errorcluster, "refnum out"=w624:T3)  [unwired: 4 in, 1 out]
      }
    }
    frame #2 {
      n365 = for {
        N: 35 -> [_]
        tunnel: w631 -> [w647]
        tunnel: [w645] -> w629
        tunnel: w630 -> [w644]
        tunnel: [w643] -> w628
        tunnel: [w633] -> w627 mode=indexing
        i -> [w636]
        w634 = 1 ("索引 (列)")
        n366 = Increment(x=w636) -> (x+1=w641:i32)
        n367 = Number To Decimal String(number=w641) -> (decimal integer string=w640:string)  [unwired: 1 in]
        n368 = Concatenate Strings("扫码关键词" ("字符串"), w640) -> (w639:string)
        n369 = call-poly <vilib>:"Read Key.vi"("section"="Setup", "error in (no error)"=w644, "key"=w639, "refnum"=w647) -> ("error out"=w643:errorcluster, "value"=w637:string, "refnum out"=w645:T3)  [unwired: 4 in, 1 out]
        n370 = property on="表格控件" class="Tbl (严格)"() -> ("Value"=w638:string[][])  [unwired: 2 in, 2 out]
        n371 = Replace Array Subset(array=w638, new element=w637, index (row)=w636, index (col)=w634) -> (w635:string[][])
        n372 = property on="表格控件" class="Tbl (严格)"("Value"=w635) -> ()  [unwired: 2 in, 2 out]
        n373 = Index Array(array=w635, index (row)=w636, index (col)=w634) -> (element=w633:string)
      }
      n374 = property on="扫码关键词" class="Ring (严格)"("Strings []"=w627) -> ()  [unwired: 2 in, 2 out]
    }
    frame #3 {
      n375 = for {
        N: 35 -> [_]
        tunnel: w652 -> [w668]
        tunnel: [w666] -> w650
        tunnel: w651 -> [w665]
        tunnel: [w664] -> w649
        tunnel: [w654] -> w648 mode=indexing
        i -> [w656]
        w655 = 2 ("索引 (列)")
        n376 = Increment(x=w656) -> (x+1=w662:i32)
        n377 = Number To Decimal String(number=w662) -> (decimal integer string=w661:string)  [unwired: 1 in]
        n378 = Concatenate Strings("产品型号" ("字符串"), w661) -> (w660:string)
        n379 = call-poly <vilib>:"Read Key.vi"("section"="Setup", "error in (no error)"=w665, "key"=w660, "refnum"=w668) -> ("error out"=w664:errorcluster, "value"=w658:string, "refnum out"=w666:T3)  [unwired: 4 in, 1 out]
        n380 = property on="表格控件" class="Tbl (严格)"() -> ("Value"=w659:string[][])  [unwired: 2 in, 2 out]
        n381 = Replace Array Subset(array=w659, new element=w658, index (row)=w656, index (col)=w655) -> (w657:string[][])
        n382 = property on="表格控件" class="Tbl (严格)"("Value"=w657) -> ()  [unwired: 2 in, 2 out]
        n383 = Index Array(array=w657, index (row)=w656, index (col)=w655) -> (element=w654:string)
      }
      n384 = property on="选择产品型号B" class="Ring (严格)"("Strings []"=w648) -> ()  [unwired: 2 in, 2 out]
      n385 = property on="选择产品型号A" class="Ring (严格)"("Strings []"=w648) -> ()  [unwired: 2 in, 2 out]
    }
    frame #4 {
      n386 = for {
        N: 35 -> [_]
        tunnel: w673 -> [w689]
        tunnel: [w687] -> w671
        tunnel: w672 -> [w686]
        tunnel: [w685] -> w670
        tunnel: [w675] -> w669 mode=indexing
        i -> [w678]
        w677 = 3 ("索引 (列)")
        n387 = Increment(x=w678) -> (x+1=w683:i32)
        n388 = Number To Decimal String(number=w683) -> (decimal integer string=w682:string)  [unwired: 1 in]
        n389 = Concatenate Strings("检验员" ("字符串"), w682) -> (w681:string)
        n390 = call-poly <vilib>:"Read Key.vi"("section"="Setup", "error in (no error)"=w686, "key"=w681, "refnum"=w689) -> ("error out"=w685:errorcluster, "value"=w679:string, "refnum out"=w687:T3)  [unwired: 4 in, 1 out]
        n391 = property on="表格控件" class="Tbl (严格)"() -> ("Value"=w680:string[][])  [unwired: 2 in, 2 out]
        n392 = Replace Array Subset(array=w680, new element=w679, index (row)=w678, index (col)=w677) -> (w676:string[][])
        n393 = property on="表格控件" class="Tbl (严格)"("Value"=w676) -> ()  [unwired: 2 in, 2 out]
        n394 = Index Array(array=w676, index (row)=w678, index (col)=w677) -> (element=w675:string)
      }
      n395 = call <vilib>:"Close Config Data.vi"("error in (no error)"=w670, "refnum"=w671) -> ()  [unwired: 8 in, 2 out]
      n396 = property on="选择检验员B" class="Ring (严格)"("Strings []"=w669) -> ()  [unwired: 2 in, 2 out]
      n397 = property on="选择检验员A" class="Ring (严格)"("Strings []"=w669) -> ()  [unwired: 2 in, 2 out]
    }
  }
  n398 = while {
    stop <- FALSE stop-if-true
    n399 = local read "启动仪器"() -> (w693:dbl)
    n400 = local write "左合格"(FALSE) -> ()
    n401 = Equal To 0?(x=w693) -> ()  [unwired: 1 out]
    n402 = call "ReadRealStatus气密机一.vi"("从站地址"=u8 255, "VISA"=refnum<visa-resource-name> "COM8", "baud rate"=u32 9600) -> ("Ready"=→"Ready":bool, "Pass"=w701:bool, "StepCode"=w698:u16, "ProgramNumber"=→"ProgramNumber":u16, "Pressure"=w696:dbl, "PressureUnit"=→"PressureUnit":u16, "AL"=w702:bool, "Leak"=w697:dbl, "PressureAL"=w703:bool, "RD"=w704:bool, "TD"=w700:bool, "StatusResults"=→"StatusResults":u16, "LeakUnit"=→"LeakUnit":u16)
    "合格" <- w701
    "StepCode" <- w698
    "实时漏率A" <- w697
    "实时压力A" <- w696
    n403 = case shown="0, 默认" w698 {
      tunnel: w697 -> [_ _ w714]
      tunnel: w696 -> [_ _ w713]
      frame 0, Default {
      }
      frame 1 {
        n404 = property on="最终结果A" class="Bool (严格)"("Colors [4]"=cluster{u32, u32}[] [{12369084, 12369084}] ("颜色[4]")) -> ()  [unwired: 2 in, 2 out]
      }
      frame 6 {
        "结果压力" <- w713
        "结果漏率" <- w714
      }
    }
    n405 = Compound Arithmetic op=OR ("复合运算")(w700, w704, w703, w702, w701) -> (w705:bool)
    n406 = case shown="0" "合格状态左" {
      tunnel: w705 -> [w715 _ w916]
      tunnel: "单腔/双腔A" -> [_ w719 _]
      tunnel: "单腔/双腔A" -> [_ w718 _]
      frame 0 {
        n407 = case shown="假" w715 {
          frame False {
            n408 = local write "合格状态左"(0.0 ("合格状态")) -> ()
          }
          frame True {
            n409 = local write "合格状态左"(1.0 ("合格状态")) -> ()
          }
        }
      }
      frame 1 {
        n410 = flat-sequence {
          tunnel: [w725] -> w722
          tunnel: [w726] -> w720
          tunnel: w719 -> [w726]
          tunnel: w718 -> [w725]
          tunnel: [w733] -> w724
          tunnel: [w732] -> w723
          tunnel: w722 -> [w732]
          tunnel: [w731] -> w721
          tunnel: w720 -> [w731]
          tunnel: w724 -> [w756]
          tunnel: w723 -> [w754]
          tunnel: w721 -> [w753]
          frame #0 {
            n411 = local write "最终结果A"(FALSE ("最终结果")) -> ()
            n412 = Increment(x="检测次数") -> (x+1=w729:u16)
            n413 = property on="最终结果A" class="Bool (严格)"("Colors [4]"=cluster{u32, u32}[] [{13816530, 13816530}] ("颜色[4]")) -> ()  [unwired: 2 in, 2 out]
            n414 = local write "检测次数"(w729) -> ()
          }
          frame #1 {
            n415 = property on="LeakUnit" class="Ring (严格)"() -> ("Value"=w734:u16)  [unwired: 2 in, 2 out]
            n416 = local read "合格"() -> (w733:bool)
            n417 = property on="PressureUnit" class="Ring (严格)"() -> ("Value"=w735:u16)  [unwired: 2 in, 2 out]
            n418 = Wait (ms)(milliseconds to wait=u32 200 ("等待时间（毫秒）")) -> ()  [unwired: 1 out]
            n419 = case shown="8000" w734 {
              frame 0, Default {
              }
              frame 1000 {
                n420 = local write "泄漏单位"("cm3/min" ("压力单位")) -> ()
              }
              frame 2000 {
                n421 = local write "泄漏单位"("ml/h" ("压力单位")) -> ()
              }
              frame 6000 {
                "泄漏单位" <- "pa"
              }
              frame 7000 {
                n422 = local write "泄漏单位"("pa") -> ()
              }
              frame 8000 {
                n423 = local write "泄漏单位"("pa/s" ("泄漏单位")) -> ()
              }
              frame 9000 {
                n424 = local write "泄漏单位"("pa/s" ("泄漏单位")) -> ()
              }
              frame 51000 {
                n425 = local write "泄漏单位"("ml/min" ("压力单位")) -> ()
              }
            }
            n426 = case shown="真" w733 {
              frame False {
                n427 = local write "结果"("NG" ("结果")) -> ()
              }
              frame True {
                n428 = Increment(x="合格次数") -> (x+1=w750:u16)
                n429 = local write "合格次数"(w750) -> ()
                "结果" <- "OK" ("结果")
              }
            }
            n430 = case shown="15000" w735 {
              frame 0, Default {
              }
              frame 11000 {
                n431 = local write "压力单位"("Bar" ("压力单位")) -> ()
              }
              frame 12000 {
                n432 = local write "压力单位"("Kpa" ("压力单位")) -> ()
              }
              frame 13000 {
                n433 = local write "压力单位"("Psi" ("压力单位")) -> ()
              }
              frame 14000 {
                n434 = local write "压力单位"("mbar" ("压力单位")) -> ()
              }
              frame 15000 {
                "压力单位" <- "Mpa"
              }
            }
          }
          frame #2 {
            n435 = local read "当前序号A"() -> (w757:string)
            n436 = local read "检测次数"() -> (w755:u16)
            n437 = local write "修改当前序号A"(w757) -> ()
            n438 = case shown="2" w755 {
              tunnel: w756 -> [_ w761 w837]
              tunnel: w754 -> [_ w759 _]
              tunnel: w753 -> [_ w758 _]
              frame 0, Default {
              }
              frame 1 {
                n439 = flat-sequence {
                  tunnel: [w763] -> w762
                  tunnel: w761 -> [w763]
                  tunnel: w762 -> [w768]
                  tunnel: [w766] -> w760
                  tunnel: w759 -> [w767]
                  tunnel: w758 -> [w766]
                  tunnel: w760 -> [w826]
                  frame #0 {
                    n440 = call "序号加一子vi.vi"() -> ("当日序号"=w764:string)  [unwired: 11 in]
                    n441 = local write "当前序号A"(w764) -> ()
                  }
                  frame #1 {
                    n442 = case shown="真" w768 {
                      tunnel: [w815 w818] -> w797
                      tunnel: [w814 w819] -> w798
                      frame False {
                        n443 = local read "实时漏率A"() -> (w813:dbl)
                        n444 = Equal To 0?(x=w813) -> (x = 0?=w812:bool)
                        n445 = case shown="真" w812 {
                          tunnel: [w816 99999.0] -> w815
                          frame False {
                            n446 = local read "实时漏率A"() -> (w816:dbl)
                          }
                          frame True {
                          }
                        }
                        n447 = local read "实时压力A"() -> (w814:dbl)
                      }
                      frame True {
                        n448 = local read "结果漏率"() -> (w818:dbl)
                        n449 = local read "结果压力"() -> (w819:dbl)
                      }
                    }
                    n450 = case shown="真" w768 {
                      tunnel: [w803 w807] -> w769
                      tunnel: w767 -> [w802 w806]
                      frame False {
                        n451 = case shown="假" w802 {
                          tunnel: ["NG" ("结果") _] -> w803
                          frame False {
                            n452 = property on="最终结果A" class="Bool (严格)"("Colors [4]"=cluster{u32, u32}[] [{16711680, 16711680}] ("颜色[4]")) -> ()  [unwired: 2 in, 2 out]
                          }
                          frame True {
                          }
                        }
                      }
                      frame True {
                        n453 = case shown="真" w806 {
                          tunnel: ["OK" ("结果") _] -> w807
                          frame False {
                            n454 = local write "最终结果A"(TRUE ("最终结果")) -> ()
                            n455 = property on="最终结果A" class="Bool (严格)"("Colors [4]"=cluster{u32, u32}[] [{6618880, 6618880}] ("颜色[4]")) -> ()  [unwired: 2 in, 2 out]
                          }
                          frame True {
                            n456 = property on="最终结果A" class="Bool (严格)"("Colors [4]"=cluster{u32, u32}[] [{13816530, 13816530}] ("颜色[4]")) -> ()  [unwired: 2 in, 2 out]
                          }
                        }
                      }
                    }
                    n457 = local read "ProgramNumber"() -> (w792:u16)
                    n458 = Number To Decimal String(number=w792, width (-)=i16 3 ("宽度(-)")) -> (decimal integer string=w793:string)
                    n459 = call <vilib>:"Space Constant.vi"() -> ("String"=w794:string)
                    n460 = Search and Replace String(replace all?=TRUE ("替换全部？(F)"), input string=w793, search string=w794, replace string="0" ("替换字符串(\"\")")) -> (number of replacements=→"替换数量":i32)  [unwired: 4 in, 3 out]
                    n461 = local read "扫码选程序"() -> (w796:bool)
                    n462 = case shown="假" w796 {
                      tunnel: [w820 w824] -> w801
                      frame False {
                        n463 = property on="选择产品型号A" class="Ring (严格)"() -> ("Strings []"=w821:string[], "Value"=w822:u16)  [unwired: 2 in, 2 out]
                        n464 = Index Array(array=w821, index=w822) -> (element=w820:string)
                      }
                      frame True {
                        n465 = local read "ATEQ程序号-1"() -> (w823:i32)
                        n466 = property on="选择产品型号A" class="Ring (严格)"() -> ("Strings []"=w825:string[])  [unwired: 2 in, 2 out]
                        n467 = Index Array(array=w825, index=w823) -> (element=w824:string)
                      }
                    }
                    n468 = local read "当前序号A"() -> (w791:string)
                    n469 = Format Date/Time String(time format string (%c)="%Y%m%d" ("时间格式字符串(%c)")) -> (date/time string=w785:string)  [unwired: 2 in]
                    n470 = local read "泄漏单位"() -> (w789:string)
                    n471 = local read "压力单位"() -> (w788:string)
                    n472 = Write to Text File(file (use dialog)=path "d:/序号.txt" ("文件（使用对话框）"), text=w791) -> ()  [unwired: 2 in, 3 out]
                    n473 = Number To Fractional String(number=w797, width (-)=i16 5 ("宽度(-)"), precision (6)=i16 2 ("精度(6)")) -> (F-format string=w787:string)  [unwired: 1 in]
                    n474 = Number To Fractional String(number=w798, width (-)=i16 6 ("宽度(-)"), precision (6)=i16 2 ("精度(6)")) -> (F-format string=w786:string)  [unwired: 1 in]
                    n475 = Concatenate Strings(w785, w791, "A" ("时间格式字符串(%c)")) -> (w799:string)
                    n476 = Format Date/Time String(time format string (%c)="%Y/%m/%d %H:%M:%S" ("时间格式字符串(%c)")) -> (date/time string=w790:string)  [unwired: 2 in]
                    n477 = Concatenate Strings(w787, w789) -> (w800:string)
                    n478 = Concatenate Strings(w786, w788) -> (w771:string)
                    n479 = local read "二维码A"() -> (w770:string)
                    n480 = Write to Text File(file (use dialog)=path "d:/检测时间.txt" ("文件（使用对话框）"), text=w790) -> ()  [unwired: 2 in, 3 out]
                    n481 = Write to Text File(file (use dialog)=path "d:/腔道1泄漏量.txt" ("文件（使用对话框）"), text=w800) -> ()  [unwired: 2 in, 3 out]
                    n482 = Write to Text File(file (use dialog)=path "d:/腔道1压力.txt" ("文件（使用对话框）"), text=w771) -> ()  [unwired: 2 in, 3 out]
                    n483 = call "数据库保存子vi.vi"("#1 Pressure"=w771, "Part No."=w801, "Result"=w769, "2D Code"=w770, "#1 Leakage"=w800, "Serial No."=w799, "Time"=w790) -> ()  [unwired: 5 in]
                  }
                  frame #2 {
                    n484 = case shown="假" w826 {
                      frame False {
                        w827 = u16 0 ("合格次数")
                        n485 = local write "检测次数"(w827) -> ()
                        n486 = local write "合格次数"(w827) -> ()
                      }
                      frame True {
                      }
                    }
                  }
                }
              }
              frame 2 {
                n487 = flat-sequence {
                  tunnel: w837 -> [w866]
                  tunnel: [w850] -> w836
                  tunnel: [w849] -> w835
                  tunnel: [w839] -> w834
                  tunnel: [w848] -> w833
                  tunnel: [w847] -> w832
                  tunnel: [w846] -> w831
                  tunnel: [w845] -> w830
                  tunnel: [w844] -> w829
                  tunnel: [w843] -> w828
                  tunnel: w836 -> [w903]
                  tunnel: w835 -> [w904]
                  tunnel: w834 -> [w901]
                  tunnel: w833 -> [w899]
                  tunnel: w832 -> [w897]
                  tunnel: w831 -> [w895]
                  tunnel: w830 -> [w893]
                  tunnel: w829 -> [w891]
                  tunnel: w828 -> [w889]
                  frame #0 {
                    n488 = case shown="真" w866 {
                      tunnel: [w884 w887] -> w873
                      tunnel: [w883 w888] -> w874
                      frame False {
                        n489 = local read "实时漏率A"() -> (w882:dbl)
                        n490 = Equal To 0?(x=w882) -> (x = 0?=w881:bool)
                        n491 = case shown="假" w881 {
                          tunnel: [w885 99999.0] -> w884
                          frame False {
                            n492 = local read "实时漏率A"() -> (w885:dbl)
                          }
                          frame True {
                          }
                        }
                        n493 = local read "实时压力A"() -> (w883:dbl)
                      }
                      frame True {
                        n494 = local read "结果漏率"() -> (w887:dbl)
                        n495 = local read "结果压力"() -> (w888:dbl)
                      }
                    }
                    n496 = local read "合格次数"() -> (w842:u16)
                    n497 = Equal?(x=w842, y=u16 2) -> (x = y?=w840:bool)
                    n498 = case shown="真" w840 {
                      tunnel: ["NG" "OK"] -> w839
                      frame False {
                        n499 = property on="最终结果A" class="Bool (严格)"("Colors [4]"=cluster{u32, u32}[] [{16711680, 16711680}] ("颜色[4]")) -> ()  [unwired: 2 in, 2 out]
                        "最终结果A" <- FALSE ("最终结果")
                      }
                      frame True {
                        w879 = TRUE ("最终结果")
                        n500 = property on="最终结果A" class="Bool (严格)"("Colors [4]"=cluster{u32, u32}[] [{6618880, 6618880}] ("颜色[4]")) -> ()  [unwired: 2 in, 2 out]
                        n501 = local write "最终结果A"(w879) -> ()
                        "左合格" <- w879
                      }
                    }
                    n502 = local read "泄漏单位"() -> (w871:string)
                    n503 = local read "压力单位"() -> (w870:string)
                    n504 = local read "当前序号A"() -> (w872:string)
                    n505 = Number To Fractional String(number=w873, width (-)=i16 5 ("宽度(-)"), precision (6)=i16 2 ("精度(6)")) -> (F-format string=w869:string)  [unwired: 1 in]
                    n506 = Number To Fractional String(number=w874, width (-)=i16 6 ("宽度(-)"), precision (6)=i16 2 ("精度(6)")) -> (F-format string=w868:string)  [unwired: 1 in]
                    n507 = Format Date/Time String(time format string (%c)="%Y%m%d" ("时间格式字符串(%c)")) -> (date/time string=w867:string)  [unwired: 2 in]
                    n508 = Concatenate Strings(w867, w872, "A" ("提示（选择或输入文件路径）")) -> (w844:string)
                    n509 = Concatenate Strings(w869, w871) -> (w845:string)
                    n510 = Concatenate Strings(w868, w870) -> (w846:string)
                    n511 = Write to Text File(file (use dialog)=path "d:/序号.txt" ("文件（使用对话框）"), text=w872) -> ()  [unwired: 2 in, 3 out]
                    n512 = call "数据库插入子vi.vi"("result"=w839, "2_Leakage"=w845, "2_Pressure"=w846, "Serial_No"=w844) -> ()  [unwired: 8 in]
                    n513 = Write to Text File(file (use dialog)=path "d:/腔道2泄漏量.txt" ("文件（使用对话框）"), text=w845) -> ()  [unwired: 2 in, 3 out]
                    n514 = Write to Text File(file (use dialog)=path "d:/腔道2压力.txt" ("文件（使用对话框）"), text=w846) -> ()  [unwired: 2 in, 3 out]
                    n515 = property on="选择产品型号A" class="Ring (严格)"() -> ("Strings []"=w853:string[], "Value"=w854:u16)  [unwired: 2 in, 2 out]
                    n516 = property on="选择检验员A" class="Ring (严格)"() -> ("Strings []"=w851:string[], "Value"=w852:u16)  [unwired: 2 in, 2 out]
                    n517 = Index Array(array=w853, index=w854) -> (element=w849:string)
                    n518 = Index Array(array=w851, index=w852) -> (element=w843:string)
                    n519 = Read from Text File(file (use dialog)=path "d:/检测时间.txt" ("文件（使用对话框）")) -> (text=w850:string)  [unwired: 3 in, 3 out]
                    n520 = Read from Text File(file (use dialog)=path "d:/腔道2压力.txt" ("文件（使用对话框）")) -> (text=w848:string)  [unwired: 3 in, 3 out]
                    n521 = Read from Text File(file (use dialog)=path "d:/腔道1泄漏量.txt" ("文件（使用对话框）")) -> (text=w847:string)  [unwired: 3 in, 3 out]
                  }
                  frame #1 {
                    n522 = call <vilib>:"Space Constant.vi"() -> ("String"=w905:string)
                    n523 = call <vilib>:"Space Constant.vi"() -> ("String"=w902:string)
                    n524 = call <vilib>:"Space Constant.vi"() -> ("String"=w898:string)
                    n525 = call <vilib>:"Space Constant.vi"() -> ("String"=w894:string)
                    n526 = call <vilib>:"Space Constant.vi"() -> ("String"=w890:string)
                    n527 = Wait (ms)(milliseconds to wait=u32 1000 ("等待时间（毫秒）")) -> ()  [unwired: 1 out]
                    n528 = Concatenate Strings(w904, w905, w903, w902, w901, "\n", w899, w898, w897, "\n", w895, w894, w893, "\n", w891, w890, w889) -> (w907:string)
                    n529 = Write to Text File(file (use dialog)=path "d:/激光打码.txt" ("文件（使用对话框）"), text=w907) -> ()  [unwired: 2 in, 3 out]
                  }
                  frame #2 {
                    w909 = u16 0 ("合格次数")
                    n530 = local write "检测次数"(w909) -> ()
                    n531 = local write "合格次数"(w909) -> ()
                  }
                }
              }
            }
          }
          frame #3 {
            n532 = call <vilib>:"Space Constant.vi"() -> ("String"=w912:string)
            n533 = local write "二维码A"(w912) -> ()
            n534 = Write to Text File(file (use dialog)=path "d:/扫码结果.txt" ("文件（使用对话框）"), text=w912) -> ()  [unwired: 2 in, 3 out]
            n535 = call "数据库读取子vi.vi"() -> ("Data"=→"显示表格":string[][])  [unwired: 11 in]
          }
          frame #4 {
            n536 = Wait (ms)(milliseconds to wait=u32 2000 ("等待时间（毫秒）")) -> ()  [unwired: 1 out]
          }
          frame #5 {
            n537 = local write "左合格"(FALSE) -> ()
          }
          frame #6 {
            n538 = local write "合格状态左"(2.0) -> ()
          }
        }
      }
      frame 2, Default {
        n539 = case shown="真" w916 {
          frame False {
            n540 = local write "合格状态左"(0.0 ("合格状态")) -> ()
          }
          frame True {
          }
        }
      }
    }
  }
  n541 = Build Array("测试时间", "序列号", "二维码", "腔道1压力", "腔道1泄漏量", "腔道2压力", "腔道2泄漏量", "结果", "产品型号" ("元素"), "检验员") -> (w45:string[])
  n542 = while {
    shift-right: [w923] -> _
    shift-left: T2."Open" -> [w924]
    shift-right: [w921] -> _
    shift-left: _ -> [w920]
    tunnel: "错误输入（无错误）" -> [w919]
    tunnel: [w918] -> w8
    stop <- w922 stop-if-true
    n543 = case shown="\"Read\"" w924 {
      tunnel: [w927 T2."Loop" T2."Loop" T2."Read" T2."Write LOFF" T2."Loop" T2."Exit" w992] -> w923
      tunnel: [_ _ _ _ _ _ TRUE FALSE] -> w922
      tunnel: [w925 w931 w954 w962 w971 w978 w985 w991] -> w921
      tunnel: w920 -> [w925 _ w954 w962 w968 w981 w985 w991]
      tunnel: w919 -> [w926 w935 w953 w961 w974 w982 w984 w990]
      tunnel: [w926 w934 w952 w960 w972 w980 w983 w990] -> w918
      frame "Init", Default {
        n544 = Unbundle By Name(w926) -> ("status"=w928:bool)
        n545 = case shown="假" w928 {
          tunnel: [T2."Loop" T2."Exit"] -> w927
          frame False {
          }
          frame True {
          }
        }
      }
      frame "Open" {
        n546 = case shown="\"Client\"" enum16{"Server", "Client"}."Client" ("类型") {
          tunnel: "192.168.2.10" ("IP") -> [_ w947]
          tunnel: w935 -> [w939 w946]
          tunnel: [w938 w945] -> w934
          tunnel: u16 9004 ("Port") -> [w941 w944]
          tunnel: [w940 w942] -> w931
          frame "Server", Default {
            n547 = call <vilib>:"TCP Listen.vi"("error in (no error)"=w939, "port"=w941) -> ("error out"=w938:errorcluster, "connection ID"=w940:refnum<k5>)  [unwired: 5 in, 3 out]
          }
          frame "Client" {
            n548 = TCP Open Connection(address=w947, remote port or service name=w944, timeout ms (60000)=1000 ("超时毫秒(60000)"), error in (no error)=w946) -> (connection ID=w942:refnum<k5>, error out=w945:errorcluster)  [unwired: 1 in]
          }
        }
      }
      frame "Write LOFF" {
        n549 = Concatenate Strings("LOFF" ("写"), "\r") -> (w950:string)
        n550 = TCP Write(connection ID=w954, data in=w950, error in (no error)=w953, 9:100 ("超时毫秒(25000)")) -> (error out=w952:errorcluster)  [unwired: 2 out]
      }
      frame "Write LON" {
        n551 = Concatenate Strings("LON" ("写"), "\r") -> (w958:string)
        n552 = TCP Write(connection ID=w962, data in=w958, error in (no error)=w961, 9:100 ("超时毫秒(25000)")) -> (error out=w960:errorcluster)  [unwired: 2 out]
      }
      frame "Read" {
        n553 = TCP Read(connection ID=w968, bytes to read=100 ("读取的字节"), error in (no error)=w974, 7:T6."Immediate" ("模式（标准）"), 9:100 ("超时毫秒(25000)")) -> (connection ID out=w971:refnum<k5>, data out=w967:string, error out=w972:errorcluster)
        n554 = String Length(string=w967) -> (length=w966:i32)
        n555 = Greater?(x=w966, y=21) -> (0:w964:bool)
        n556 = case shown="真" w964 {
          tunnel: w967 -> [_ w977]
          frame False {
          }
          frame True {
            n557 = local write "二维码A"(w977) -> ()
            n558 = shared-variable "我的电脑\\OPC.lvlib\\左扫码合格"(TRUE ("左扫码合格")) -> ()  [unwired: 1 in, 1 out]
          }
        }
      }
      frame "Close" {
        n559 = TCP Close Connection(connection ID=w981, error in (no error)=w982) -> (connection ID out=w978:refnum<k5>, error out=w980:errorcluster)  [unwired: 1 in]
      }
      frame "Exit" {
        n560 = TCP Close Connection(connection ID=w985, error in (no error)=w984) -> (error out=w983:errorcluster)  [unwired: 1 in, 1 out]
      }
      frame "Loop" {
        (unwired) 100
        n561 = case shown="真" "左扫码启动" {
          tunnel: [_ T2."Write LON"] -> w992
          frame False {
          }
          frame True {
          }
        }
      }
    }
  }
  "错误输出 3" <- w8
  n562 = property on="显示表格" class="Tbl (严格)"("Number of Rows"=u32 25 ("行数"), "Number of Columns"=u32 8 ("列数"), "Row Headers[]"=w43, "Column Headers[]"=w45, "Height"=u32 605 ("大小:高度"), "Width"=u32 1100 ("大小:宽度")) -> ("Number of Rows"=w33:u32, "Number of Columns"=w30:u32, "Value"=w35:string[][])  [unwired: 2 in, 2 out]
  n563 = while {
    shift-right: [w999] -> _
    shift-left: T2."Open" -> [w1000]
    shift-right: [w997] -> _
    shift-left: _ -> [w996]
    tunnel: "错误输入（无错误） 2" -> [w995]
    tunnel: [w994] -> w7
    stop <- w998 stop-if-true
    n564 = case shown="\"Read\"" w1000 {
      tunnel: [w1003 T2."Loop" T2."Loop" T2."Read" T2."Write LOFF" T2."Loop" T2."Exit" w1068] -> w999
      tunnel: [_ _ _ _ _ _ TRUE FALSE] -> w998
      tunnel: [w1001 w1007 w1030 w1038 w1047 w1054 w1061 w1067] -> w997
      tunnel: w996 -> [w1001 _ w1030 w1038 w1044 w1057 w1061 w1067]
      tunnel: w995 -> [w1002 w1011 w1029 w1037 w1050 w1058 w1060 w1066]
      tunnel: [w1002 w1010 w1028 w1036 w1048 w1056 w1059 w1066] -> w994
      frame "Init", Default {
        n565 = Unbundle By Name(w1002) -> ("status"=w1004:bool)
        n566 = case shown="假" w1004 {
          tunnel: [T2."Loop" T2."Exit"] -> w1003
          frame False {
          }
          frame True {
          }
        }
      }
      frame "Open" {
        n567 = case shown="\"Client\"" enum16{"Server", "Client"}."Client" ("类型") {
          tunnel: "192.168.2.20" ("IP") -> [_ w1023]
          tunnel: w1011 -> [w1015 w1022]
          tunnel: [w1014 w1021] -> w1010
          tunnel: u16 9004 ("Port") -> [w1017 w1020]
          tunnel: [w1016 w1018] -> w1007
          frame "Server", Default {
            n568 = call <vilib>:"TCP Listen.vi"("error in (no error)"=w1015, "port"=w1017) -> ("error out"=w1014:errorcluster, "connection ID"=w1016:refnum<k5>)  [unwired: 5 in, 3 out]
          }
          frame "Client" {
            n569 = TCP Open Connection(address=w1023, remote port or service name=w1020, timeout ms (60000)=1000 ("超时毫秒(60000)"), error in (no error)=w1022) -> (connection ID=w1018:refnum<k5>, error out=w1021:errorcluster)  [unwired: 1 in]
          }
        }
      }
      frame "Write LOFF" {
        n570 = Concatenate Strings("LOFF" ("写"), "\r") -> (w1026:string)
        n571 = TCP Write(connection ID=w1030, data in=w1026, error in (no error)=w1029, 9:100 ("超时毫秒(25000)")) -> (error out=w1028:errorcluster)  [unwired: 2 out]
      }
      frame "Write LON" {
        n572 = Concatenate Strings("LON" ("写"), "\r") -> (w1034:string)
        n573 = TCP Write(connection ID=w1038, data in=w1034, error in (no error)=w1037, 9:100 ("超时毫秒(25000)")) -> (error out=w1036:errorcluster)  [unwired: 2 out]
      }
      frame "Read" {
        n574 = TCP Read(connection ID=w1044, bytes to read=100 ("读取的字节"), error in (no error)=w1050, 7:T6."Immediate" ("模式（标准）"), 9:100 ("超时毫秒(25000)")) -> (connection ID out=w1047:refnum<k5>, data out=w1043:string, error out=w1048:errorcluster)
        n575 = String Length(string=w1043) -> (length=w1042:i32)
        n576 = Greater?(x=w1042, y=21) -> (0:w1040:bool)
        n577 = case shown="真" w1040 {
          tunnel: w1043 -> [_ w1053]
          frame False {
          }
          frame True {
            n578 = local write "二维码B"(w1053) -> ()
            n579 = shared-variable "我的电脑\\OPC.lvlib\\右工位扫码合格"(TRUE ("右工位扫码合格")) -> ()  [unwired: 1 in, 1 out]
          }
        }
      }
      frame "Close" {
        n580 = TCP Close Connection(connection ID=w1057, error in (no error)=w1058) -> (connection ID out=w1054:refnum<k5>, error out=w1056:errorcluster)  [unwired: 1 in]
      }
      frame "Exit" {
        n581 = TCP Close Connection(connection ID=w1061, error in (no error)=w1060) -> (error out=w1059:errorcluster)  [unwired: 1 in, 1 out]
      }
      frame "Loop" {
        (unwired) 100
        n582 = case shown="假" "右扫码启动" {
          tunnel: [_ T2."Write LON"] -> w1068
          frame False {
          }
          frame True {
          }
        }
      }
    }
  }
  "错误输出 4" <- w7
  n583 = shared-variable "我的电脑\\OPC.lvlib\\左扫码合格"(w3) -> ()  [unwired: 1 in, 1 out]
  n584 = Array Size(array=w35) -> (size(s)=w34:i32[])
  n585 = shared-variable "我的电脑\\OPC.lvlib\\右工位扫码合格"(w3) -> ()  [unwired: 1 in, 1 out]
  n586 = Index Array(array=w34) -> (element #1=w32:i32, element #2=w31:i32)  [unwired: 2 in]
  n587 = Max & Min(x=w33, y=w32) -> (max(x,y)=w29:u32)  [unwired: 1 out]
  n588 = Max & Min(x=w30, y=w31) -> (max(x,y)=w28:u32)  [unwired: 1 out]
  n589 = Read from Text File(file (use dialog)=path "d:/序号.txt" ("文件（使用对话框）")) -> (text=w39:string)  [unwired: 3 in, 3 out]
  n590 = for {
    N: w29 -> [_]
    tunnel: w28 -> [w1073]
    tunnel: u32 16448250 -> [w1072]
    tunnel: u32 13816530 -> [w1071]
    i -> [w1070]
    n591 = for {
      N: w1073 -> [_]
      tunnel: w1070 -> [w1083]
      tunnel: w1072 -> [w1077]
      tunnel: w1071 -> [w1076]
      tunnel: w1070 -> [w1074]
      i -> [w1082]
      n592 = Quotient & Remainder(x=w1074, y=u32 2) -> (x-y*floor(x/y)=w1080:u32)  [unwired: 1 out]
      n593 = Equal?(x=w1080, y=u32 0) -> (x = y?=w1078:bool)
      n594 = Select(t=w1077, s=w1078, f=w1076) -> (s? t:f=w1075:u32)
      n595 = Bundle By Name(cluster="活动单元格:活动单元格", "Row"=w1083, "Column"=w1082) -> (w1084:T1)
      n596 = property on="显示表格" class="Tbl (严格)"("Active Cell"=w1084, "Cell BG Color"=w1075) -> ()  [unwired: 2 in, 2 out]
    }
  }
  n597 = local write "修改当前序号A"(w39) -> ()
  n598 = local write "当前序号A"(w39) -> ()
  n599 = local write "二维码A"("") -> ()
  n600 = local write "二维码B"("") -> ()
  n601 = while {
    stop <- FALSE stop-if-true
    n602 = Wait (ms)(milliseconds to wait=u32 100 ("等待时间（毫秒）")) -> ()  [unwired: 1 out]
  }
